vi "AlliGator Calibration Actions.vi"(0 "AlliGator Q Elements":T4[](array[typedef]), 1 "VI in":refnum<vi>, 2 "Script in":bool, 5 "data value reference":refnum<data-value>, 7 "AlliGator Q Event in":T5=enum."GUI:Idle", 9 "Data":variant, 11 "error in (no error)":errorcluster, 12 "AlliGator Ctrl Refnums":T6) -> (3 "Script out":bool, 4 "Alligator Queue Element 1 (+ 2)":T4[](array[typedef]), 6 "AlliGator IV DVR":refnum<data-value>, 10 "[Notebook Message]":T1[](array[typedef]) {"Message Style"."Text Alignment" items=["Left", "Right", "Center"]}, 15 "error out":errorcluster)   [LabVIEW 2021, in "AlliGator Action Engine.lvlib"]
doc: "Processes AlliGator phasor calibration-related actions."
uses:
  AlliGator Action Engine.lvlib
  AlliGator Internal Variables v2.ctl
  <vilib>/vision/Image Controls.llb/IMAQ Image.ctl
  AlliGator Gate Image Set.ctl
  AlliGator FLI Dataset Type.ctl
  AlliGator Data Series Type.ctl
  AlliGator Dataset Channel.ctl
  AlliGator Gate Arithmetic.ctl
  AlliGator Displayed Image.ctl
  Image/Named ROI Description.ctl
  AlliGator Decay Metadata v3.ctl
  AlliGator Decay Background Subtraction Info.ctl
  AlliGator Baseline Subtraction Method.ctl
  Graphs/XY Graph/XY Graph Plot Shift Parameters.ctl
  Graphs/XY Graph/XY Graph Plot Shift Method.ctl
  AlliGator Decay Extrapolation Parameters.ctl
  Phasor/Calibration Phasor (m, phi).ctl
  Phasor/Phasor Reference Series.ctl
  Phasor/Phasor Calibration Map v2.ctl
  Phasor/Phasor (g, s).ctl
  AlliGator Raw Phasor Plot Data v4.ctl
  Phasor/Phasor Standard Deviation Options.ctl
  AlliGator Phasor Multi-Harmonic Data.ctl
  Phasor/Phasor Harmonic Data.ctl
  AlliGator Decay Fit Options & Parameters v2.ctl
  Fits/IRF(X)PSED/Decay Fit Options v2.ctl
  Fits/Decay Convolution/Decay Model.ctl
  Fits/Residual Type.ctl
  Fits/IRF(X)PSED/Fit Weights Type.ctl
  Fits/Non-linear Fitting Method v2.ctl
  Fits/Fit Calculation Method.ctl
  Fits/Non-linear Fitting Algorithm.ctl
  AlliGator Decay Fit Parameter Constraints 2.ctl
  Fits/IRF(X)PSED/Decay Fit Parameters In List.ctl
  Fits/IRF(X)PSED/MLE Baseline Offset Type.ctl
  AlliGator Decay Preprocessing Parameters.ctl
  Fits/IRF(X)PSED/Decay Fit Parameters & Derived Quantities List.ctl
  AlliGator Q Event.ctl
  AlliGator Ctrl Refnums.ctl
  AlliGator Other Ctrl Refnums.ctl
  AlliGator State Indicator.ctl
  AlliGator Phasor Plot Ctrl Refnums.ctl
  AlliGator Phasor Graph Ctrl Refnums.ctl
  Phasor/Phasor Calibration Type.ctl
  AlliGator Dataset Ctrl Refnums.ctl
  AlliGator Registered Events Ctrl Refnums.ctl
  AlliGator Image Histogram Control Refnums.ctl
  Histograms/Linear Histogram Options.ctl
  Histograms/Histogram Bin Option.ctl
  Histograms/Histogram Bin Position.ctl
  AlliGator Decay Fit Map Control Refnums.ctl
  AlliGator Q Element.ctl
  Notebook/Notebook Message Object.ctl
  Rich Text Box/Text Formatting.ctl
  Rich Text Box/Text Colors.ctl
  Alligator Elements Order in Action Stack.ctl
  AlliGator State Indicators List.ctl
  Graphs/XY Graph/XY Graph Mouse Click Event Data.ctl
  Graphs/XY Graph/XY Graph Refnum.ctl
  <vilib>/Utility/miscctls.llb/LVPoint32TypeDef.ctl
  Files/Load-Save File Info.ctl
  c3660eb9-da68-4ace-825a-127935e87b4e.vi
  Variant/Variant to Data/Variant to I32.vi
  Variant/Variant to Data/Variant to Boolean.vi
  AlliGator Add Single Action to Stack.vi
  Graphs/Get Plot at Mouse Click (XY Graph)/Get Plot at Mouse Click [AAC].vi
  AlliGator Add Action Array to Stack.vi
  AlliGator Scripts.lvlib
  GUI/GUI.lvlib
  Phasor/Phasor.lvlib
  AlliGator Settings.lvlib
  AlliGator Phasor Calibration.lvlib
  Files/Files.lvlib
  AlliGator GUI.lvlib
  Rich Text Box/Rich Text Box.lvlib
  Graphs/XY Graph/XY Graph Add-Ons.lvlib
  Graphs/Graphs.lvlib
  AlliGator Phasor Graph.lvlib
  Variant/Variant to Data/Variant to Data.lvlib
  AlliGator Internal Variables.lvlib
  Sound/Sound.lvlib
  AlliGator Source Image.lvlib
  AlliGator Decay Fit Parameter Map.lvlib
  Image/Image.lvlib
  AlliGator Decay Preprocessing.lvlib
  AlliGator Files.lvlib
  AlliGator Phasor Plot.lvlib
  Fits/Fits.lvlib
  AlliGator Decay Fit.lvlib
  AlliGator Dual-Channel Datasets.lvlib
  Histograms/Histogram Window.lvlib
  Notebook/Notebook.lvlib
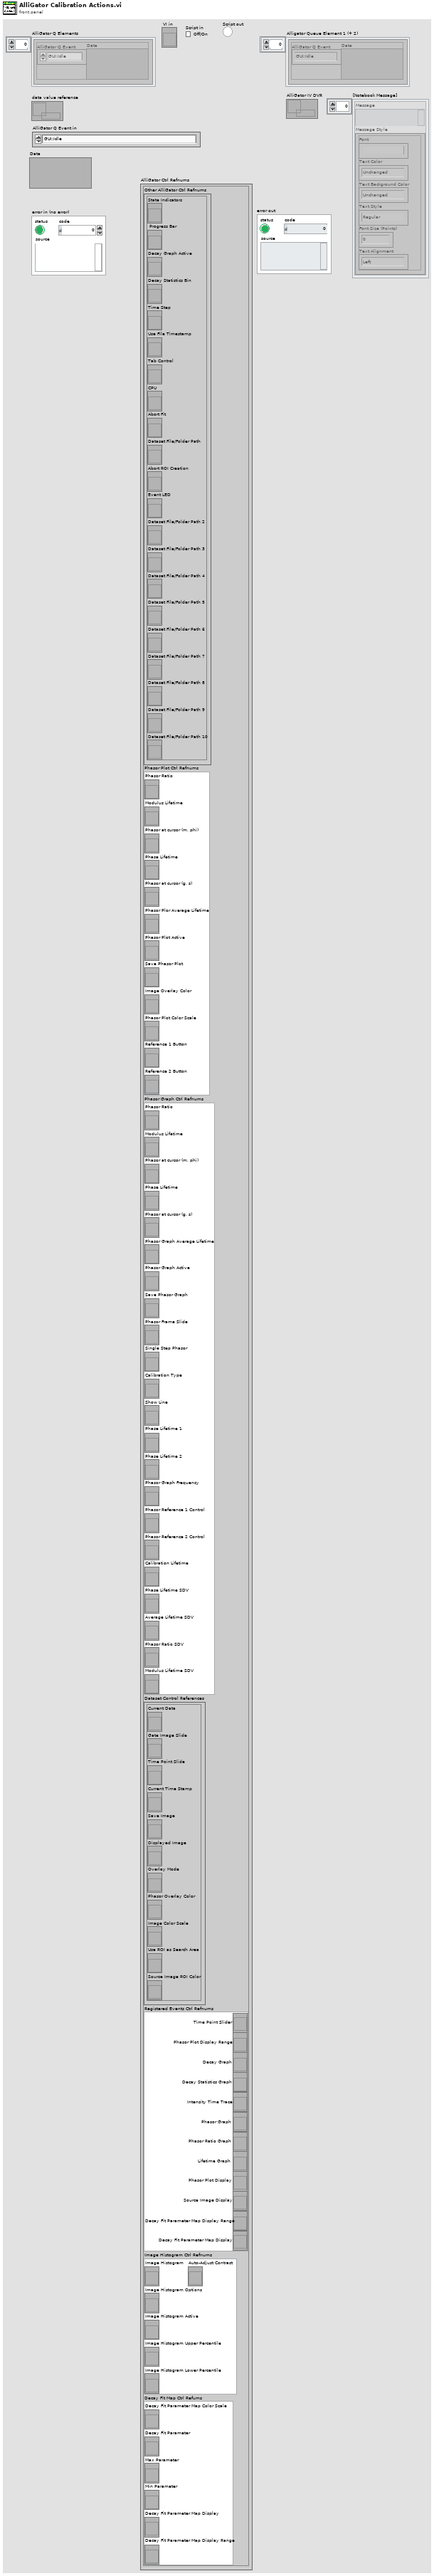
[diagram p1: front panel]
types:
  T1 = typedef "Notebook.lvlib/Notebook Message Object.ctl" = cluster{"Message":string, "Message Style":T2}
  T2 = typedef "Rich Text Box.lvlib/Text Formatting.ctl" = cluster{"Font":string, "Text Color":T3, "Text Background Color":T3, "Text Style":enum16{"Regular", "Bold", "Italic", "Underline", "Strikeout"}, "Font Size (Points)":dbl, "Text Alignment":i32}
  T3 = typedef "Rich Text Box.lvlib/Text Colors.ctl" = enum16{"Unchanged", "Black", "Blue", "Brown", "Gray", "Green", "Orange", "Pink", "Red", "White"}
  T4 = typedef "AlliGator Action Engine.lvlib/AlliGator Q Element.ctl" = cluster{"AlliGator Q Event":T5, "Data":variant}
  T5 = typedef "AlliGator Action Engine.lvlib/AlliGator Q Event.ctl" = enum16{"---- Files ----", "Files:Set Batch Export Files To Save", "Files:Set Dataset Loading & Pre-processing Options", "Files:Check #Frames in Dataset", "Files:Increment Frame Index", "Files:Open Mask Image", "Files:Open White Light Image", "Files:Open Single Dataset", "Files:New Folder of Folders Selected", "Files:Load File (all Types)_Scriptable", "Files:Move Flattened Series to Folders Series", "Files:Select Folder", "Files:Load FLI Dataset", "Files:Load Swiss SPAD 1 Dataset", "Files:Load Swiss SPAD 2 Dataset", "Files:Load .sdt FLI Dataset", "Files:Load .ptu FLI Dataset", "Files:Load .bin FLI Dataset", "Files:Load Single Gate Image Folder", "Files:Load I/m/phi Dataset (deprecated)", "Files:Load Single Image", "Files:Subtract Background File", "Files:Export FLI Dataset", "Files:Load HDF5 FLI Dataset", "Files:Set Destination File Path", "Files:Save Mask Image", "Files:Batch Conversion", "Files:New Folder Selected", "Files:Close FLI Dataset", "Files:Close FLI Dataset Series", "Files:Close White Light Image", "Files:Close Mask Image", "---- FLI Dataset ----", "FLI Dataset:Channel Arithmetic", "FLI Dataset:Export Average Lifetime Map as ASCII", "FLI Dataset:Export User-Defined Quantity Map as ASCII", "FLI Dataset:Python Function FLI Dataset Event", "FLI Dataset:ROI Analysis", "FLI Dataset:Tilted Logistic Square Gated IRF Characteristics Map", "FLI Dataset:Logistic Square Gated IRF Characteristics Map", "FLI Dataset:Square Gated IRF Characteristics Map", "FLI Dataset:Multi-ROI Single-Pixel Phasor Analysis", "FLI Dataset:Multi-ROI Single-Pixel NLSF Analysis", "FLI Dataset:All ROIs IRF Extraction", "FLI Dataset:All ROIs Decay Fit Non-Interactive (Fast + Individual IRF)", "FLI Dataset:All ROIs Phasor Analysis", "FLI Dataset:All ROIs Decay Fit", "FLI Dataset:Fluorescence Decay Statistics", "FLI Dataset:Update Decay Statistics Graph", "FLI Dataset:Get Decay from ROI", "FLI Dataset:All ROIs Average Lifetimes", "---- FLI Dataset Series ----", "FLI Dataset Series:Sum All Datasets in Series", "FLI Dataset Series:Add Dataset to Accumulated Dataset", "FLI Dataset Series:Display Accumulated Dataset", "FLI Dataset Series:Clear Dataset Series Sum", "FLI Dataset Series:Time-Series Analysis (NLSF)", "FLI Dataset Series:Time-Series Analysis (Phasor)", "---- Image ----", "Image:Update Image Profile Plots", "Image:Image Histogram Cursor Move", "Image:Image Histogram", "Image:Image Contrast", "Image:Set Image Histogram Cursor Move Flag", "Image:Clear Image Overlay", "Image:Use ROI as Search Area", "Image:Set ROI Diameter", "Image:Save Image Data as TIFF", "Image:Save Displayed Image with Overlay", "Image:Save Image Overlay Only", "Image:Save Image as Hot Pixel Mask", "Image:Change Source Image Color Palette", "Image:Copy Image to Clipboard", "Image:Source Image ROI Selection", "Image:Delete All ROIs", "Image:Delete All Unselected ROIs", "Image:Delete ROI", "Image:Merge All ROIs", "Image:Store ROI", "Image:Source Image ROI Storage", "Image:Export ROI Description to Notebook", "Image:Save ROI", "Image:Load ROI", "Image:Paste ROI Definition", "Image:Clear ROI", "Image:Identify ROIs in Mask Image", "Image:Create Complementary ROI", "Image:Create Contour ROI", "Image:Create ROI(s) from Pixels with Peak above Min_Scriptable", "Image:Create ROI(s) from Pixels with Intensity above Min_Scriptable", "Image:Compute ROI Statistics", "Image:Delete ROI(s) based on ROI Characteristics", "Image:Create ROI Grid", "Image:ROI to Individual Pixel ROIs", "Image:Python Function Source Image Event", "Image:Show Phasor Calibration Map ROI Centers", "Image:Convert ROI to Mask Image", "Image:Mouse Move", "Image:Mouse Up", "Image:Set Source Image Mouse Move Flag", "Image:Add Scale Bar Overlay", "Image:Delete Existing ROIs Option", "---- Decay ----", "Decay:Clear IRF/Reference Plot", "Decay:Clear Local IRFs", "Decay:Add Decay to Graph", "Decay:Smoothen Plot", "Decay:Smoothen Plot Tail", "Decay:Average Selected Plots", "Decay:Extract IRF", "Decay:Optimal IRF Extraction", "Decay:Threshold IRF", "Decay:Fit to Model IRF", "Decay:Fit IRF to Square Gate", "Decay:Fit IRF to Logistic Square Gate", "Decay:Fit IRF to Tilted Logistic Square Gate", "Decay:Create Bounding Cursors Set", "Decay:Export Bounding Cursors Definition to Notebook", "Decay:Denoise Plot", "Decay:Compute Cumulative Function", "Decay:Use as Reference Decay", "Decay:Show Reference Decay/IRF", "Decay:Extrapolate Decay", "Decay:Create Head & Tail Bounding Cursors", "Decay:Store Cursor-defined Head & Tail Fractions", "Decay:Rebin Plot", "Decay:1-Normalize Decay", "Decay:[0-1]-Normalize Plot", "Decay:Straighten Decay", "Decay:Shift Decay", "Decay:Fold Decay", "Decay:Fit Decay", "Decay:Global Fit of Selected Decays", "Decay:Post Global Fit Script", "Decay:Add Global Fit Parameters to Graph", "Decay:Add Decay Parameter(s) to Plot (Graph)", "Decay:Export Decay to Phasor Graph", "Decay:Plot Decay Shifts", "Decay:Compute Average Lifetime", "Decay:Plot Convolution", "Decay:Graph Tip Strip Update", "---- Decay Statistics ----", "Decay Statistics:Tip Strip Update", "---- Intensity Time Trace ----", "Intensity Time Trace:Use File Timestamp", "Intensity Time Trace:Load Intensity Corrections File", "Intensity Time Trace:Clear Intensity Corrections File", "Intensity Time Trace:Tip Strip Update", "---- Phasor Plot ----", "Phasor Plot:Build Phasor Plot", "Phasor Plot:Change Phasor Plot Color Palette", "Phasor Plot:Adjust Phasor Plot Display Range", "Phasor Plot:Highlight Image ROI in Phasor Plot", "Phasor Plot:Save Phasor Plot Image with Overlay", "Phasor Plot:Export Complex Phasor Map", "Phasor Plot:Export Phasor Ratio Map", "Phasor Plot:Export Average Lifetime Map", "Phasor Plot:Compute Phase Lifetime Histogram", "Phasor Plot:Compute Phasor Ratio Histogram", "Phasor Plot:Compute Phase Lifetime vs Intensity Scatter Plot", "Phasor Plot:Weber 2-Component Decomposition", "Phasor Plot:Update Phasor Color Map Vertices", "Phasor Plot:Clear Phasor Overlay", "Phasor Plot:Use Segment Extremities as References", "Phasor Plot:Use UC/Segment Intersections as References", "Phasor Plot:Use UC/Principal Axis Intersections as References", "Phasor Plot:Use UC/Linear Fit Intersections as References", "Phasor Plot:Update Phasor Plot Reference", "Phasor Plot:Show Local Phasor Info in Phasor Plot", "Phasor Plot:Update Phasor Plot State", "Phasor Plot:Phasor Plot ROI Storage", "Phasor Plot:Phasor Plot ROI Selection", "Phasor Plot:Python Function Phasor Plot Event", "Phasor Plot:Overlay Phasor ROI, Ratio or Map in Source Image", "Phasor Plot:Compute Decay of Selected Phasors", "Phasor Plot:Phasor at Image Pixel", "Phasor Plot:Mouse Move", "Phasor Plot:Mouse Up", "Phasor Plot:Display Range Mouse Move", "Phasor Plot:Set Mouse Move Flag", "---- Phasor Graph ----", "Phasor Graph:Calibrated Phasor Map Series", "Phasor Graph:Whole Image Phasor Scatter Plot (Todo)", "Phasor Graph:Get Phasor Value", "Phasor Graph:Create New Phasor Plot Dialog", "Phasor Graph:Update Last Phasor Value", "Phasor Graph:Update Phasor (m, phi)", "Phasor Graph:Remove Single Phasor from Plot", "Phasor Graph:Add Single Phasor to Plot", "Phasor Graph:Remove Phasor Plot", "Phasor Graph:Remove Selected Phasor Plots", "Phasor Graph:Clear Phasor Data", "Phasor Graph:Clear Phasor Graph", "Phasor Graph:Cursor Move", "Phasor Graph:Draw Cursor Connecting Line", "Phasor Graph:Clear Cursor Connecting Line", "Phasor Graph:Find UC Intersection", "Phasor Graph:Use UC/Cursor-Defined Line Intersections", "Phasor Graph:Use Selected Plots Fitted Line/UC Intersections", "Phasor Graph:Use Selected Plots Principal Axis/UC Intersections", "Phasor Graph:Show Single Phasor", "Phasor Graph:Save Single Phasor Plot", "Phasor Graph:Save All Phasor Plots", "Phasor Graph:Load Phasor Plot(s)", "Phasor Graph:Phasor Multiplication", "Phasor Graph:Compute Average Phasor", "Phasor Graph:Compute Multiple Average Phasors (Selected Plots)", "Phasor Graph:Export Single Phasor Plot Phase Lifetimes", "Phasor Graph:Phase Lifetime Trajectory", "Phasor Graph:Phase Lifetime vs Intensity Scatter Plot (deprecated)", "Phasor Graph:Parameter 2 vs Parameter 1 Scatter Plot", "Phasor Graph:Use Cursor n Location", "Phasor Graph:Set Reference n to Current Phase Lifetime Value", "Phasor Graph:Set Reference n to Lifetime Value", "Phasor Graph:Set Cursor n Location", "Phasor Graph:Save Phasor Graph Image", "Phasor Graph:Update SEPL Plot", "Phasor Graph:Export Single Phasor Plot Data", "Phasor Graph:Export Selected Phasor Plots Data", "Phasor Graph:Python Function Phasor Graph Event", "Phasor Graph:Tip Strip Update", "---- Calibration ----", "Calibration:Set Calibration Type", "Calibration:Load/Save Phasor Calibration", "Calibration:Load/Save Phasor Calibration Series", "Calibration:Load/Save Phasor Calibration Map", "Calibration:Use as Calibration", "Calibration:Compute Optimal Calibration from Phasor References", "Calibration:Clear Phasor Calibration", "Calibration:Single Phasor Calibration Information", "Calibration:Use as Calibration Series", "Calibration:Use as Calibration Map", "Calibration:Clear Calibration Series", "Calibration:Phasor Calibration Series Information", "Calibration:Clear Calibration Map", "Calibration:Phasor Calibration Map Information", "Calibration:Apply Phasor Calibration", "Calibration:Update Single Plot Calibration", "Calibration:Update Multiple Plots Calibration", "Calibration:Clear Single Plot Calibration", "Calibration:Clear All Plots Calibrations", "Calibration:Clear Plot(s) Calibration(s)?", "Calibration:Phasor Calibration Maps (# Gates Series)", "---- Phasor Ratio ----", "Phasor Ratio:Clear Reference n", "Phasor Ratio:Toggle Selected Plot(s)  Lock to Reference 1", "Phasor Ratio:Use as Reference n", "Phasor Ratio:Send Reference n to Notebook", "Phasor Ratio:Toggle Selected Plot(s)  Lock to Reference 2", "Phasor Ratio:Compute Phasor Ratio at Mouse Location", "Phasor Ratio:Compute Phasor Plot's Average Phasor Ratio", "Phasor Ratio:Compute Time-Series Phasor Ratios", "Phasor Ratio:Fit Line to Phasor Ratio Plot", "Phasor Ratio:Save References", "Phasor Ratio:Load References", "Phasor Ratio:Update Phasor Reference 1", "Phasor Ratio:Update Phasor Reference 2", "Phasor Ratio:Move Cursor n to Reference n", "Phasor Ratio:Use as Phasor Reference 1 Lifetime", "Phasor Ratio:Use as Phasor Reference 2 Lifetime", "Phasor Ratio:Export Phasor Ratio Map as ASCII", "Phasor Ratio:Tip Strip Update", "---- Lifetime & Other Parameters Graph ----", "Lifetime:Tip Strip Update", "---- Decay Fit Parameter Map ----", "Decay Fit Parameter Map:Export ROI NLSF Data as ASCII", "Decay Fit Parameter Map:Set Decay Fit  Parameter Map Selection", "Decay Fit Parameter Map:Build Decay Fit Parameter Map", "Decay Fit Parameter Map:Change Decay Fit Parameter Map Color Palette", "Decay Fit Parameter Map:Export Decay Fit Parameter Map Data as ASCII", "Decay Fit Parameter Map:Export All Decay Fit Parameter Maps Data as ASCII", "Decay Fit Parameter Map:Send Map Data to Lifetime Graph", "Decay Fit Parameter Map:Save Decay Fit Parameter Map Image", "Decay Fit Parameter Map:Save-Load IRFs & Fit Data", "Decay Fit Parameter Map:Update Local Decay Plots", "Decay Fit Parameter Map:Python Function Decay Fit Parameters Map Event", "Decay Fit Parameter Map:Overlay Decay Fit Parameter Map in Source Image", "Decay Fit Parameter Map:Plot Map Data vs Intensity", "Decay Fit Parameter Map:Mouse Up", "Decay Fit Parameter Map:Display Range Mouse Move", "---- Generic Graph ----", "Generic Graph:Generic XY Graph Event", "Generic Graph:Python Function XY Graph Event", "Generic Graph:New Plot", "Generic Graph:Save Plot", "Generic Graph:XY Plot Histogram", "Generic Graph:Set XY Graph Plot Name", "Generic Graph:Set Last Cursor Style", "Generic Graph:Tip Strip Update", "---- GUI ----", "GUI:Start Script", "GUI:Type of Displayed Image Changed", "GUI:Gate Image Slide Changed", "GUI:Show Busy Icon", "GUI:Show Busy Icon & Abort Button", "GUI:Hide Busy Icon", "GUI:Hide Busy Icon & Abort Button", "GUI:Abort", "GUI:End Script", "GUI:Start Timing", "GUI:End Timing", "GUI:Set State Indicator", "GUI:Send Parameters JSON Strings to Clipboard", "GUI:Set Gate Step", "GUI:Idle", "GUI:Initialization", "GUI:Quit", "GUI:Increment Dataset Index", "GUI:Set Dataset Index to -1", "GUI:Time Series Slider Moved", "GUI:Time Series Slider Changed", "GUI:Toggle Playback or Loop", "GUI:Playback Script", "GUI:Set Phasor Frequency", "GUI:Open Window", "GUI:Start Test Script", "GUI:End Test Script", "DEBUG"}
  T6 = typedef "AlliGator GUI.lvlib/AlliGator Ctrl Refnums.ctl" = cluster{"Other AlliGator Ctrl Refnums":T7, "Phasor Plot Ctrl Refnums":T8, "Phasor Graph Ctrl Refnums":T9, "Dataset Control References":T10, "Registered Events Ctrl Refnums":T11, "Image Histogram Ctrl Refnums":T12, "Decay Fit Map Ctrl Refums":T13}
  T7 = typedef "AlliGator GUI.lvlib/AlliGator Other Ctrl Refnums.ctl" = cluster{"State Indicators":refnum<vi>, " Progress Bar":refnum<vi>, "Decay Graph Active":refnum<vi>, "Decay Statistics Bin":refnum<vi>, "Time Step":refnum<vi>, "Use File Timestamp":refnum<vi>, "Tab Control":refnum<vi>, "CPU":refnum<vi>, "Abort Fit":refnum<vi>, "Dataset File/Folder Path":refnum<vi>, "Abort ROI Creation":refnum<vi>, "Event LED":refnum<vi>, "Dataset File/Folder Path 2":refnum<vi>, "Dataset File/Folder Path 3":refnum<vi>, "Dataset File/Folder Path 4":refnum<vi>, "Dataset File/Folder Path 5":refnum<vi>, "Dataset File/Folder Path 6":refnum<vi>, "Dataset File/Folder Path 7":refnum<vi>, "Dataset File/Folder Path 8":refnum<vi>, "Dataset File/Folder Path 9":refnum<vi>, "Dataset File/Folder Path 10":refnum<vi>}
  T8 = typedef "AlliGator GUI.lvlib/AlliGator Phasor Plot Ctrl Refnums.ctl" = cluster{"Phasor Ratio":refnum<vi>, "Modulus Lifetime":refnum<vi>, "Phasor at cursor (m, phi)":refnum<vi>, "Phase Lifetime":refnum<vi>, "Phasor at cursor (g, s)":refnum<vi>, "Phasor Plor Average Lifetime":refnum<vi>, "Phasor Plot Active":refnum<vi>, "Save Phasor Plot":refnum<vi>, "Image Overlay Color":refnum<vi>, "Phasor Plot Color Scale":refnum<vi>, "Reference 1 Button":refnum<vi>, "Reference 2 Button":refnum<vi>}
  T9 = typedef "AlliGator GUI.lvlib/AlliGator Phasor Graph Ctrl Refnums.ctl" = cluster{"Phasor Ratio":refnum<vi>, "Modulus Lifetime":refnum<vi>, "Phasor at cursor (m, phi)":refnum<vi>, "Phase Lifetime":refnum<vi>, "Phasor at cursor (g, s)":refnum<vi>, "Phasor Graph Average Lifetime":refnum<vi>, "Phasor Graph Active":refnum<vi>, "Save Phasor Graph":refnum<vi>, "Phasor Frame Slide":refnum<vi>, "Single Step Phasor":refnum<vi>, "Calibration Type":refnum<vi>, "Show Line":refnum<vi>, "Phase Lifetime 1":refnum<vi>, "Phase Lifetime 2":refnum<vi>, "Phasor Graph Frequency":refnum<vi>, "Phasor Reference 1 Control":refnum<vi>, "Phasor Reference 2 Control":refnum<vi>, "Calibration Lifetime":refnum<vi>, "Phase Lifetime SDV":refnum<vi>, "Average Lifetime SDV":refnum<vi>, "Phasor Ratio SDV":refnum<vi>, "Modulus Lifetime SDV":refnum<vi>}
  T10 = typedef "AlliGator GUI.lvlib/AlliGator Dataset Ctrl Refnums.ctl" = cluster{"Current Data":refnum<vi>, "Gate Image Slide":refnum<vi>, "Time Point Slide":refnum<vi>, "Current Time Stamp":refnum<vi>, "Save Image":refnum<vi>, "Displayed Image":refnum<vi>, "Overlay Mode":refnum<vi>, "Phasor Overlay Color":refnum<vi>, "Image Color Scale":refnum<vi>, "Use ROI as Search Area":refnum<vi>, "Source Image ROI Color":refnum<vi>}
  T11 = typedef "AlliGator GUI.lvlib/AlliGator Registered Events Ctrl Refnums.ctl" = cluster{"Time Point Slider":refnum<vi>, "Phasor Plot Display Range":refnum<vi>, "Decay Graph":refnum<vi>, "Decay Statistics Graph":refnum<vi>, "Intensity Time Trace":refnum<vi>, "Phasor Graph":refnum<vi>, "Phasor Ratio Graph":refnum<vi>, "Lifetime Graph":refnum<vi>, "Phasor Plot Display":refnum<vi>, "Source Image Display":refnum<vi>, "Decay Fit Parameter Map Display Range":refnum<vi>, "Decay Fit Parameter Map Display":refnum<vi>}
  T12 = typedef "AlliGator GUI.lvlib/AlliGator Image Histogram Control Refnums.ctl" = cluster{"Image Histogram":refnum<vi>, "Image Histogram Options":refnum<vi>, "Image Histogram Active":refnum<vi>, "Image Histogram Upper Percentile":refnum<vi>, "Image Histogram Lower Percentile":refnum<vi>, "Auto-Adjust Contrast":refnum<vi>}
  T13 = typedef "AlliGator Decay Fit Parameter Map.lvlib/AlliGator Decay Fit Map Control Refnums.ctl" = cluster{"Decay Fit Parameter Map Color Scale":refnum<vi>, "Decay Fit Parameter":refnum<vi>, "Max Parameter":refnum<vi>, "Min Parameter":refnum<vi>, "Decay Fit Parameter Map Display":refnum<vi>, "Decay Fit Parameter Map Display Range":refnum<vi>}
  T14 = typedef "AlliGator Action Engine.lvlib/Alligator Elements Order in Action Stack.ctl" = enum16{"Enqueue 2 AFTER 1", "Enqueue 2 BEFORE 1"}
  T15 = typedef "AlliGator Action Engine.lvlib/AlliGator State Indicators List.ctl" = enum16{"Phasor Calibration Defined", "Phasor Calibration Series Defined", "Phasor Calibration Map Defined", "Phasor Reference 1 Defined", "Phasor Reference 2 Defined", "Lifetime Reference 1 Defined", "Lifetime Reference 2 Defined", "Phasor Calibration Used", "Phasor Calibration Series Used", "Phasor Calibration Map Used", "Dataset Update Needed", "Phasor Plot Update Needed", "Reference/IRF Defined", "Individual IRFs Defined"}
  T16 = typedef "Phasor.lvlib/Phasor Calibration Map v2.ctl" = cluster{"Phasor Frequency":dbl[unit], "Calibration Lifetime":dbl[unit], "ROI Centers":cluster{"X":i32, "Y":i32}[], "ROI Descriptors":T17[], "Map Resolution X":i32, "Map Resolution Y":i32, "z Array":cdb[]}
  T17 = typedef "ROI Descriptor" = cluster{"Global Rectangle":i32[], "Contours":cluster{"ID":enum32{"External", "Internal"}, "Type":u32, "Coordinates":i32[]}[]}
  T18 = typedef "Phasor.lvlib/Phasor Reference Series.ctl" = cluster{"m Array":dbl[], "phi Array":dbl[], "Phasor Frequency":dbl[unit], "Calibration Lifetime":dbl[unit]}
  T19 = typedef "Phasor.lvlib/Calibration Phasor (m, phi).ctl" = cluster{"m":dbl, "phi":dbl, "Phasor Frequency":dbl[unit], "Reference Lifetime":dbl[unit]}
  T20 = typedef "XY Graph Add-Ons.lvlib/XY Graph Mouse Click Event Data.ctl" = cluster{"Multiplot XY Graph":T21, "Mouse Coordinates":T22}
  T21 = typedef "XY Graph Add-Ons.lvlib/XY Graph Refnum.ctl" = refnum<vi>
  T22 = typedef "LVPoint32TypeDef.ctl" = cluster{"Horizontal":i32, "Vertical":i32}
  T23 = typedef "Files.lvlib/Load-Save File Info.ctl" = cluster{"Load/Save":bool, "File Path":path}
  T24 = typedef "Phasor.lvlib/Phasor Calibration Type.ctl" = enum16{"None", "Single Phasor", "Phasor Series", "Phasor Map"}
  T25 = typedef "Phasor.lvlib/Phasor (g, s).ctl" = cluster{"g":dbl, "s":dbl}
  T26 = typedef "AlliGator Internal Variables.lvlib/AlliGator Internal Variables v2.ctl" = cluster{"Displayed Image":T27, "White Light Image":T27, "Mask Image":T27, "ROI Mask Image":T27, "Current Dataset Images 1":T28, "Background Dataset Images 1":T28, "Current Dataset Images 2":T28, "Background Dataset Images 2":T28, "Current Dataset Arithmetic Images":T28, "Accumulated Dataset Images 1":T28, "Accumulated Dataset Images 2":T28, "Accumulated Dataset Arithmetic Images":T28, "Phasor Plot Image":T27, "Decay Fit Parameter Map Image":T27, "Single Data Point Path":path, "White Light Image Path":path, "Mask Image Path":path, "Time-Series Folder":path, "[Time-Series Paths]":path[], "Current Dataset":i32, "Single Dataset Type":T29, "Current Folder":string, "AlliGator Data Series Type":T30, "# Datasets":i32, "Dual-Channel Dataset":bool, "Selected Channel Name":string, "Dataset Channel":T31, "Channel Arithmetic":T32, "Dual-Channel Background Dataset":bool, "Background Channel":T31, "Dual-Channel Accumulated Dataset":bool, "Start Time":dbl, "[Time-Series Timestamps]":dbl[], "[Intensity Corrections]":dbl[], "Time Series Script":bool, "Type of Displayed Image":T33, "Gate Image Slide":u16, "# Gates":i32, "ROIs":T34[], "ROI Decay":cluster{"t Array":dbl[], "I Array":dbl[]}, "Valid Decay":bool, "Decay  Metadata":T35, "Reference Decay Plot Name":string, "Reference Decay":cluster{"t Array":dbl[], "I Array":dbl[]}, "Decay Shift Plot":cluster{"Time Stamps":dbl[], "Decay Shifts":dbl[]}, "[Decays Max Values]":sgl[], "[Decays Min Values]":sgl[], "Calibration Phasor":T19, "Calibration Phasor Series":T18, "Phasor Calibration Map":T16, "Calibration Map MD5 Digest":string, "Last Raw Phasor":T25, "Last Calibrated Phasor":T25, "Last Calibrated Phasor SDV":T25, "Phasor Graph:Phasor Plot":cluster{"g Array":dbl[], "s Array":dbl[]}, "Phasor Graph:Phasor SDV Plot":cluster{"g Array":dbl[], "s Array":dbl[]}, "[Phasor Graph:Raw Phasor Plots]":T41[], "Phasor Plot locked to Ref 1":i32, "[Phasor Plot(s) locked to Ref 1]":i32[], "[Phasor Plot(s) locked to Ref 2]":i32[], "[Pixel Phasors]":T25[], "[[Sum Image]]":dbl[][], "[[CSG Phasors]]":csg[][], "[[Valid Pixel?]]":bool[][], "I/m/phi Dataset":cluster{"I/m/phi Dataset?":bool, "Base Frequency":dbl[unit], "Harmonic Orders":u8[]}, "Multi Phasor Plot Data":T43, "Decay Fit Options & Parameters":T45, "Fit Options: Decay Preprocessing Parameters":T56, "Fit Options: Reference Decay":cluster{"t Array":dbl[], "I Array":dbl[]}, "Is Full Image Parameters Map":bool, "Is Single-Pixels Parameters Map":bool, "NLSF Parameters Map X Resolution":i32, "NLSF Parameters Map Y Resolution":i32, "[Single Decay Fit Parameters]":dbl[], "Fit Model":T47, "[[Multiple Decays Fit Parameters]]":dbl[][], "[[Multiple Decays Fit Parameter SDVs]]":dbl[][], "[[IRFs]]":dbl[][], "IRF Array Time Axis":dbl[], "Decay Array Time Axis":dbl[], "[Decay Fit Parameter Names]":T57[], "[[Phasor Ratios]]":dbl[][], "[[Average Lifetimes]]":dbl[][], "Amplitude Weighted Average Lifetime":bool, "[Decay Sum]":dbl[], "[[User-defined Quantities]]":dbl[][], "User-defined Quantity":string}
  T27 = typedef "IMAQ Image.ctl" = refnum<image>
  T28 = typedef "AlliGator Internal Variables.lvlib/AlliGator Gate Image Set.ctl" = cluster{"SGL Image Max":T27, "SGL Image Sum":T27, "SGL Gate Images":T27[], "SGL Image Min":T27}
  T29 = typedef "AlliGator Files.lvlib/AlliGator FLI Dataset Type.ctl" = enum16{"HDF5 FLI Dataset", "Gate Image Folder", ".sdt FLI Dataset (Becker & Hickl)", ".ptu FLI Dataset (PicoQuant)", "SS1 FLI Dataset", "SS2 FLI Dataset", "I/m/phi Dataset", ".bin FLI Dataset (PicoQuant Binned)", ".bin FLI Dataset (Piccolo Binned)"}
  T30 = typedef "AlliGator Files.lvlib/AlliGator Data Series Type.ctl" = enum16{"Not a Supported Series", "Gate Images Folder Series", "SwissSPAD 2 Dataset Series", "B&H FLI Dataset Series", "PicoQuant PTU FLI Dataset Series", "PicoQuant BIN FLI Dataset Series", "Piccolo hist BIN FLI Dataset Series", "HDF5 FLI Dataset Series"}
  T31 = typedef "AlliGator Dual-Channel Datasets.lvlib/AlliGator Dataset Channel.ctl" = enum16{"G2", "INT"}
  T32 = typedef "AlliGator Settings.lvlib/AlliGator Gate Arithmetic.ctl" = enum16{"None", "INT-G2", "G2/INT*<INT>", "(1 - G2/INT)*<INT>"}
  T33 = typedef "AlliGator Source Image.lvlib/AlliGator Displayed Image.ctl" = enum16{"Single Gate", "Sum of All Gates", "Max of All Gates", "Min of All Gates", "-", "White Ligth Image", "Mask Image"}
  T34 = typedef "Image.lvlib/Named ROI Description.ctl" = cluster{"ROI Descriptor":T17, "ROI Name":string, "Overlay Color":u32}
  T35 = typedef "AlliGator Phasor Graph.lvlib/AlliGator Decay Metadata v3.ctl" = cluster{"ROI Descriptor":T17, "ROI Center":cluster{"X":i32, "Y":i32}, "Decay Background Subtraction Info":T36, "Decay Reverted":bool, "Decay Smoothened":bool, "Decay Straightened":bool, "Fitted Tau (Decay Straightening)":dbl, "Decay Shift Parameters":T38, "Decay Shifted":bool, "Decay Extrapolated":bool, "Decay Extrapolation Parameters":T40, "Decay Normalized":bool, "Fold Decay":bool, "# Folds":u32}
  T36 = typedef "AlliGator Decay Analysis.lvlib/AlliGator Decay Preprocessing.lvlib/AlliGator Decay Background Subtraction Info.ctl" = cluster{"Laser Period":dbl[unit], "Gate Duration":dbl[unit], "Baseline Subtraction Method":T37, "Background Definition Range":cluster{"Min Gate":dbl[unit], "Max Gate":dbl[unit]}, "Total Intensity w/o Bkgd Subtraction":dbl, "Bkgd-subtracted Intensity (exp)":dbl, "# Data Points":i32, "Background/Gate":dbl, "Fitted Lifetime":dbl[unit], "Bkgd-subtracted Intensity (theo)":dbl}
  T37 = typedef "AlliGator Decay Analysis.lvlib/AlliGator Decay Preprocessing.lvlib/AlliGator Baseline Subtraction Method.ctl" = enum16{"Mean", "Min", "Square Gated Single-Exponential", "File", "Constant"}
  T38 = typedef "XY Graph Add-Ons.lvlib/XY Graph Plot Shift Parameters.ctl" = cluster{"Type":T39, "Shift":dbl[unit], "Threshold":dbl, "Rotate":bool}
  T39 = typedef "XY Graph Add-Ons.lvlib/XY Graph Plot Shift Method.ctl" = enum16{"Default", "CFD", "Threshold", "Cross-Correlation"}
  T40 = typedef "AlliGator Decay Analysis.lvlib/AlliGator Decay Preprocessing.lvlib/AlliGator Decay Extrapolation Parameters.ctl" = cluster{"Additional Points":u32, "Head Fraction":dbl, "Fitted Tau":dbl, "Use Periodicity":bool, "Use Cursors":bool, "Tail Fraction":dbl}
  T41 = typedef "AlliGator Phasor Graph.lvlib/AlliGator Raw Phasor Plot Data v4.ctl" = cluster{"Phasor Plot Name":string, "Raw Phasor Plot":T25[], "Phasor Frequency":dbl[unit], "[Decay Metadata]":T35[], "Raw Phasor Plot SDV":T25[], "Phasor SDV Options":T42, "[Calibration Phasor]":T19[]}
  T42 = typedef "Phasor.lvlib/Phasor Standard Deviation Options.ctl" = cluster{"Compute Estimated SDV":bool, "# Replicas":u32, "Use Estimated Average Phasor":bool}
  T43 = typedef "AlliGator Phasor Plot.lvlib/AlliGator Phasor Multi-Harmonic Data.ctl" = cluster{"Base Frequency":dbl[unit], "# Harmonics":u8, "Harmonic Orders":u8[], "Phasor Plot Settings Checksum":u64, "Phasor Harmonic Data Array":T44[]}
  T44 = typedef "Phasor.lvlib/Phasor Harmonic Data.ctl" = cluster{"Phasor Harmonic Name":string, "Phasor Plot Settings Checksum":u64, "Phasor Frequency":dbl[unit], "Base Frequency":dbl[unit], "Harmonic Order":u8, "Phasor Plot Parameters":string, "Phasor Array [[CSG]]":csg[][], "Dataset File Path":path}
  T45 = typedef "AlliGator Decay Fit Parameter Map.lvlib/AlliGator Decay Fit Options & Parameters v2.ctl" = cluster{"SYNC Period":dbl[unit], "Fit Options":T46, "Fit Parameter Constraints":T53[], "MLE Baseline Offset":dbl, "MLE Baseline Offset Type":T55}
  T46 = typedef "Fits.lvlib/Decay Fit Options v2.ctl" = cluster{"Show Fit Residuals":bool, "Fit Model":T47, "Residual Type":T48, "Max Decay Percentile":dbl, "Min Decay Percentile":dbl, "Show Full Decay":bool, "Weights":T49, "Fitting Method":T50, "Compute Parameter Uncertainties":bool, "Periodic Boundaries":bool, "Model Calculation":T51, "Period":dbl[unit], "Termination Criteria":cluster{"Max Iterations":i32, "Max Function Calls":i32, "Max Time":dbl[unit], "Function Tolerance":dbl, "Parameter Tolerance":dbl, "Gradient Tolerance":dbl, "Min Lambda":dbl, "Max Lambda":dbl, "Initial Tick Count":u32}, "Offset Resolution":dbl[unit], "Use Local IRF":bool, "Fitting Algorithm":T52}
  T47 = typedef "Fits.lvlib/Decay Model.ctl" = enum16{"1-Exponential", "2-Exponentials"}
  T48 = typedef "Fits.lvlib/Residual Type.ctl" = enum16{"Standard", "Normalized", "Reduced"}
  T49 = typedef "Fits.lvlib/Fit Weights Type.ctl" = enum16{"Unweighted", "1/Variance", "Best of All"}
  T50 = typedef "Fits.lvlib/Non-linear Fitting Method v2.ctl" = enum16{"Least Square", "Least Absolute Residual", "Bisquare", "MLE", "-", "Best of All"}
  T51 = typedef "Fits.lvlib/Fit Calculation Method.ctl" = enum16{"Simulation", "Convolution", "Integration"}
  T52 = typedef "Fits.lvlib/Non-linear Fitting Algorithm.ctl" = enum16{"Levenberg-Marquardt", "Trust-Region Dogleg"}
  T53 = typedef "AlliGator Decay Analysis.lvlib/AlliGator Decay Fit.lvlib/AlliGator Decay Fit Parameter Constraints 2.ctl" = cluster{"Fit Parameter":T54, "Min Value":dbl, "Max Value":dbl, "Global":bool, "Used":bool}
  T54 = typedef "Fits.lvlib/Decay Fit Parameters In List.ctl" = enum16{"Offset", "Baseline", "A_1", "tau_1", "A_2", "tau_2"}
  T55 = typedef "Fits.lvlib/MLE Baseline Offset Type.ctl" = enum32{"Absolute", "Percentage"}
  T56 = typedef "AlliGator Decay Analysis.lvlib/AlliGator Decay Preprocessing.lvlib/AlliGator Decay Preprocessing Parameters.ctl" = cluster{"Background Subtraction":bool, "Straighten Decay":bool, "Reverse Gates":bool, "1-Normalized Decay":bool, "Smoothen Decay":bool, "Smoothing Parameter":dbl, "Shift Decay":bool, "Decay Shift Parameters":T38, "Extrapolate Decay":bool, "Additional Points":u32, "Head Fraction":dbl, "Pixel-Normalize Decay":bool, "Use Periodicity":bool, "Use Cursors":bool, "Tail Fraction":dbl, "Use Decay Pre-Processing":bool, "Fold Decay":bool, "# Folds":u32, "[0-1]-Normalized Decay":bool}
  T57 = typedef "Fits.lvlib/Decay Fit Parameters & Derived Quantities List.ctl" = enum16{"Offset", "Baseline", "A_1", "tau_1", "A_2", "tau_2", "<tau>_a", "f1_a", "f2_a", "<tau>_i", "f1_i", "f2_i", "-", "R^2", "Chi^2"}
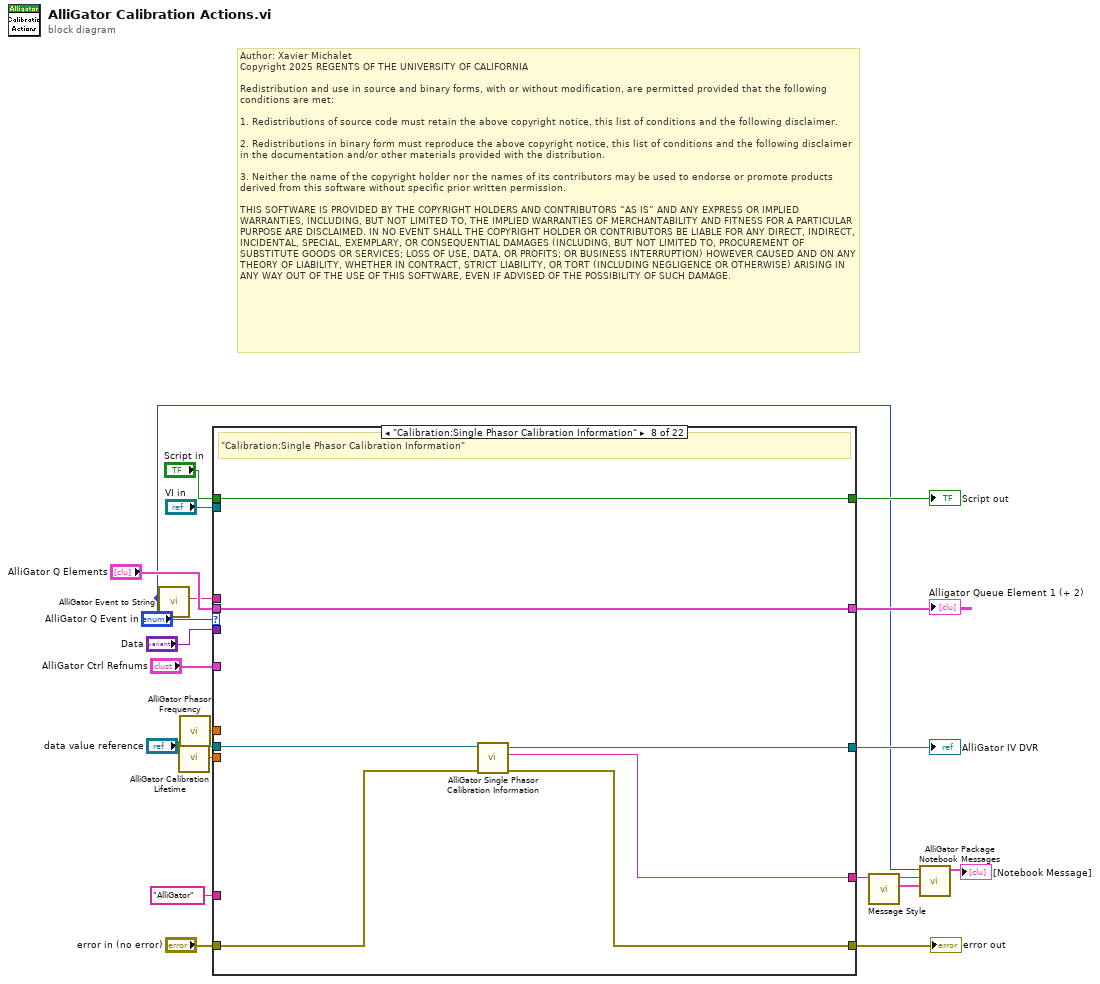
[diagram p0: block diagram]
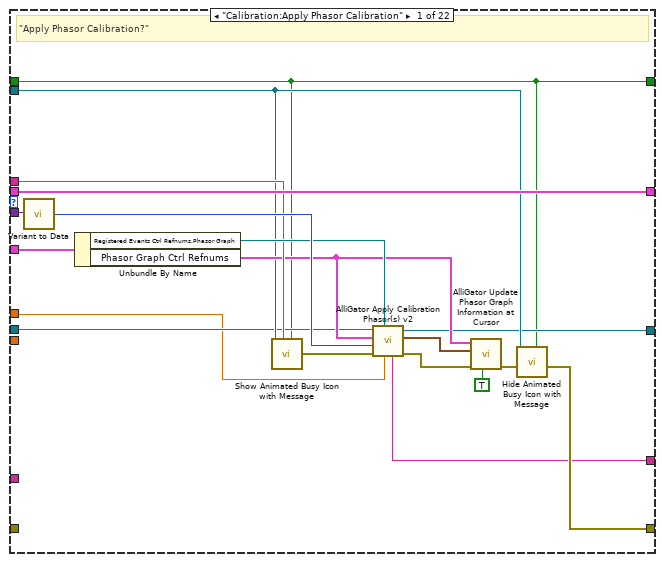
[diagram p2: hidden frame]
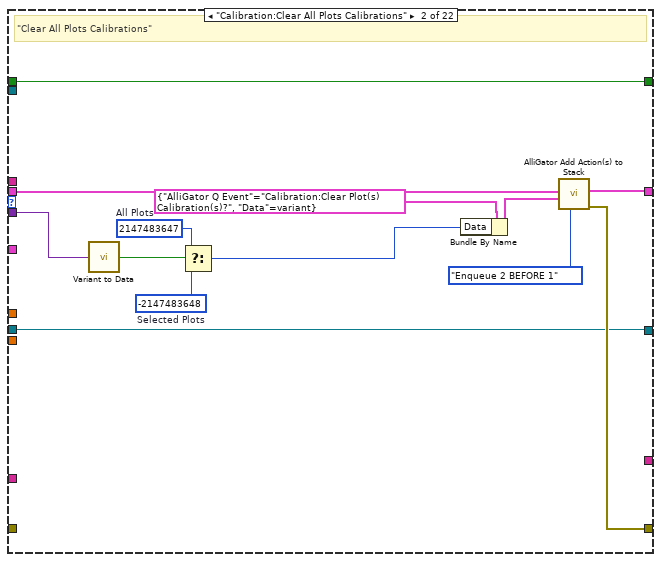
[diagram p3: hidden frame]
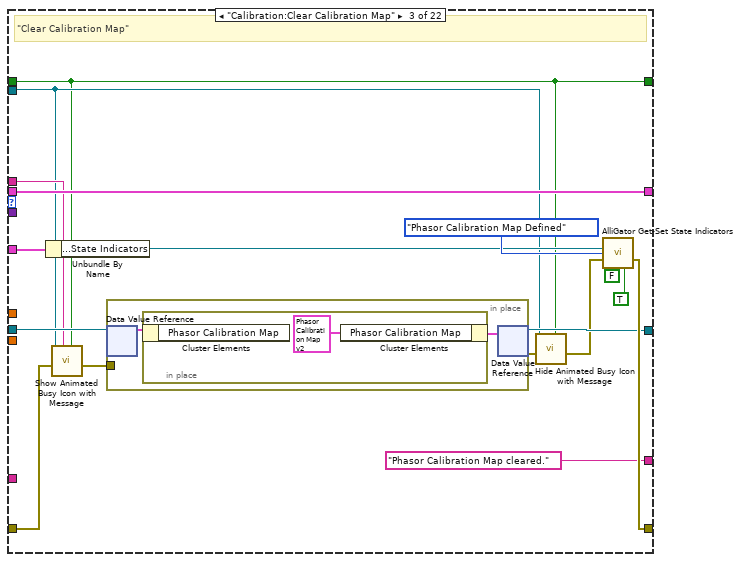
[diagram p4: hidden frame]
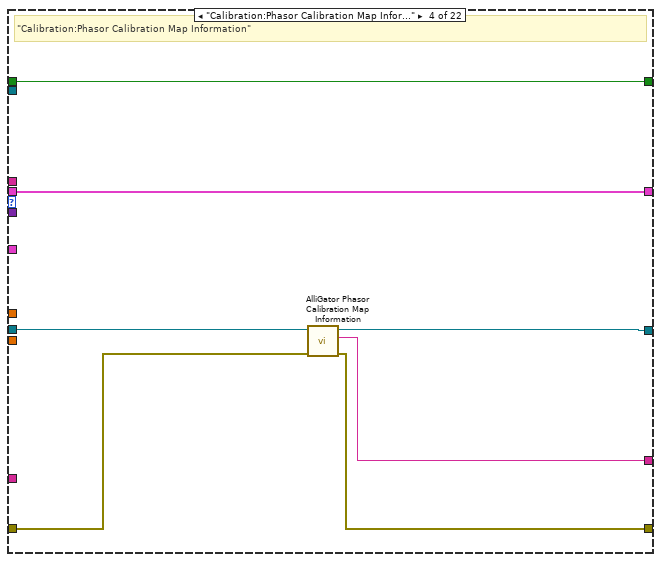
[diagram p5: hidden frame]
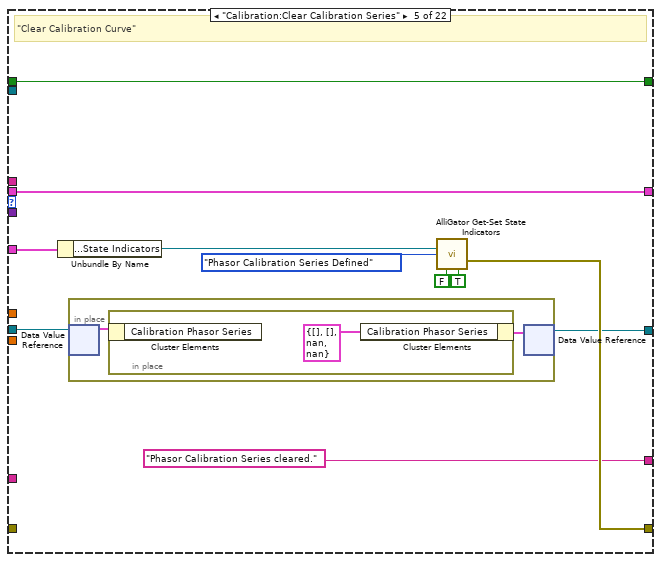
[diagram p6: hidden frame]
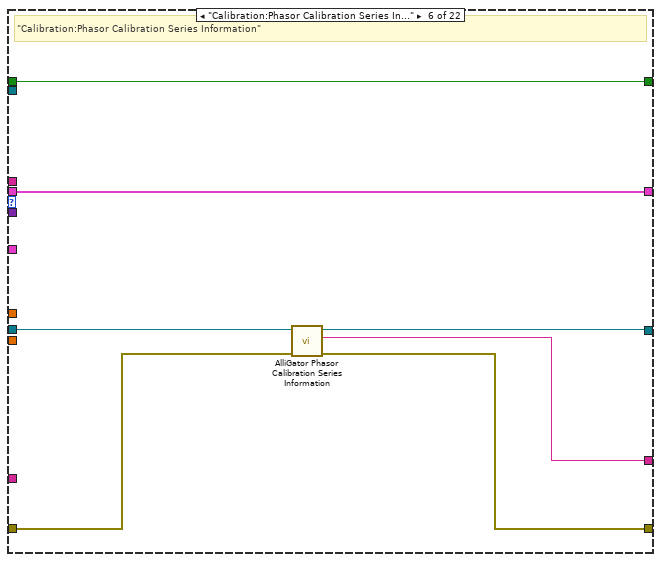
[diagram p7: hidden frame]
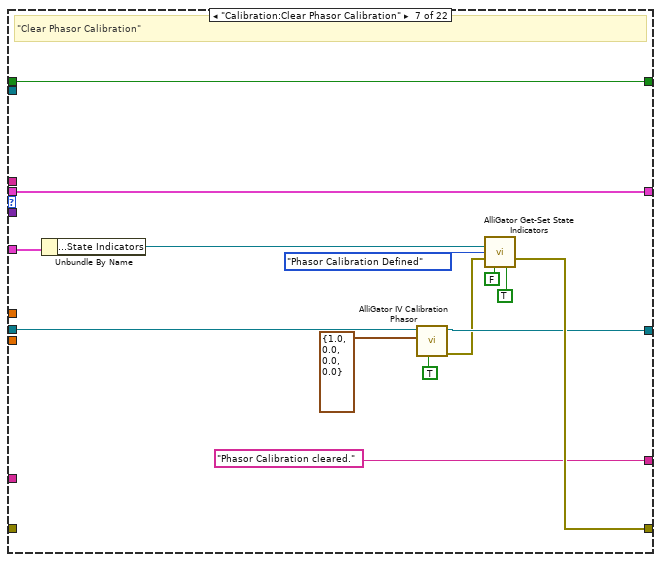
[diagram p8: hidden frame]
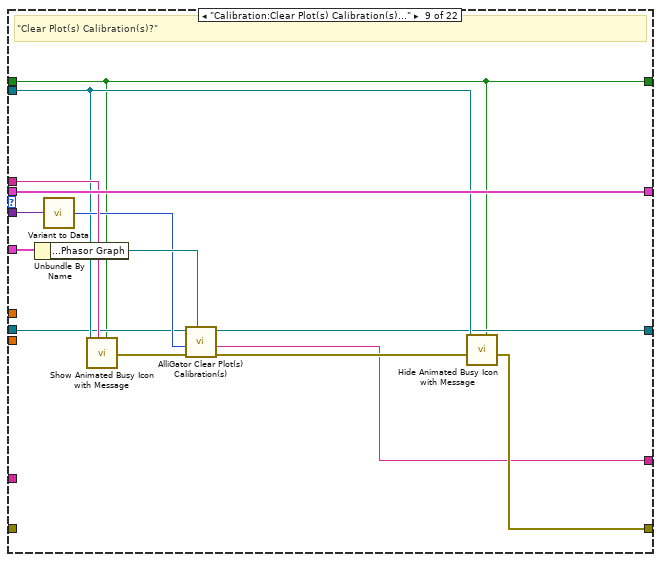
[diagram p9: hidden frame]
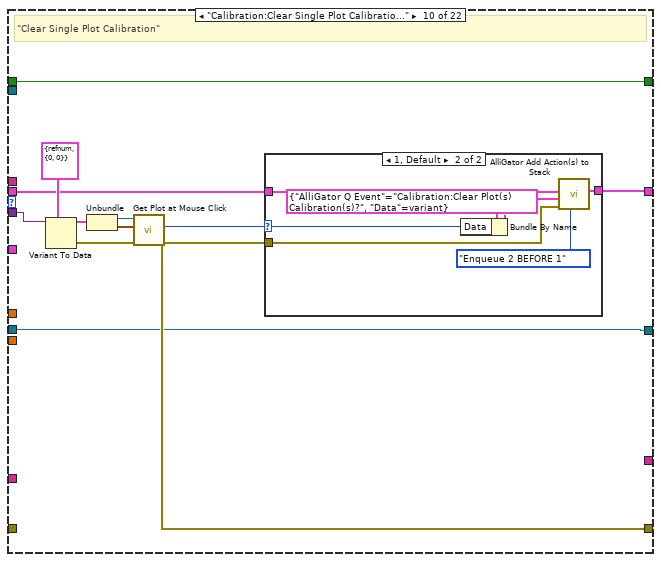
[diagram p10: hidden frame]
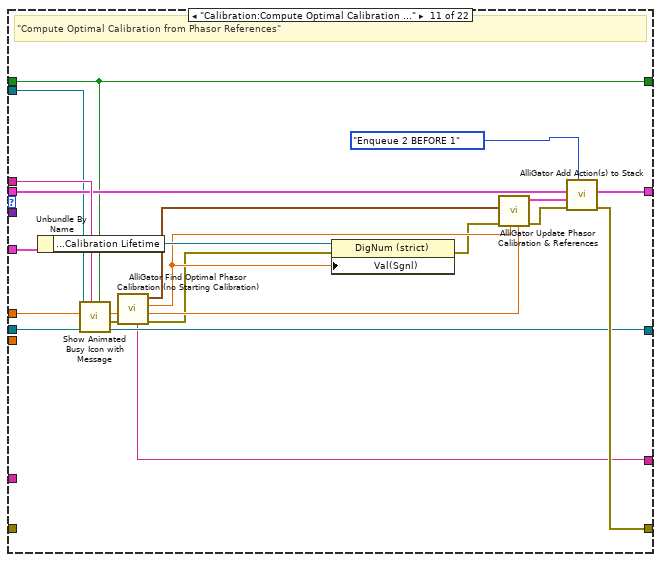
[diagram p12: hidden frame]
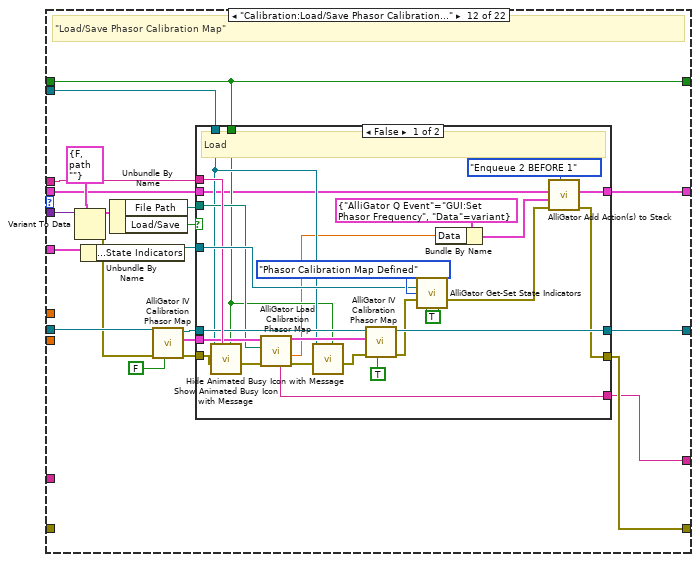
[diagram p13: hidden frame]
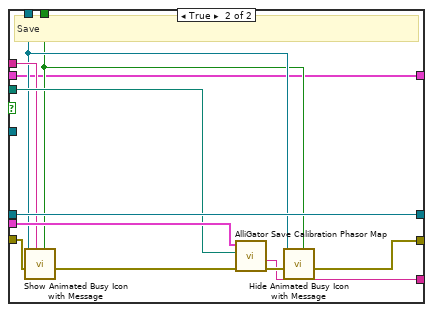
[diagram p14: hidden frame]
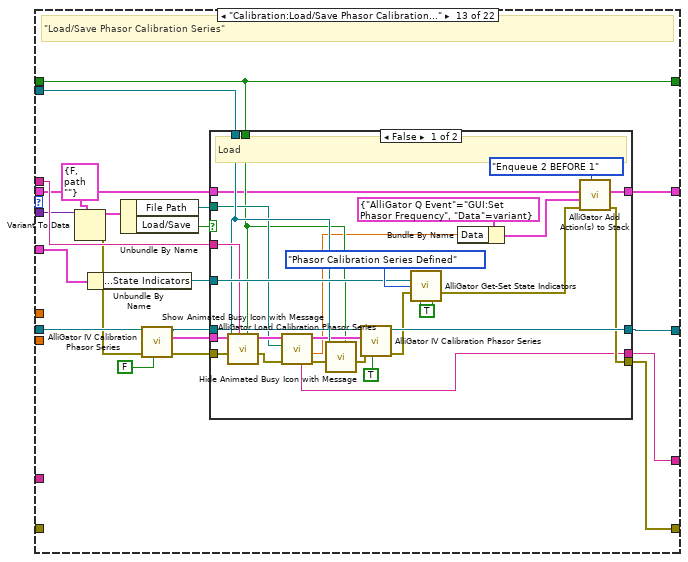
[diagram p15: hidden frame]
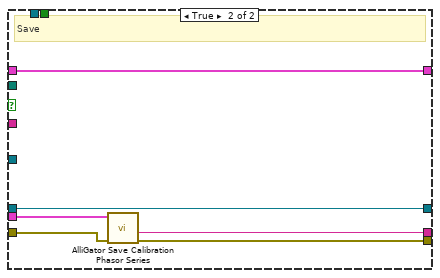
[diagram p16: hidden frame]
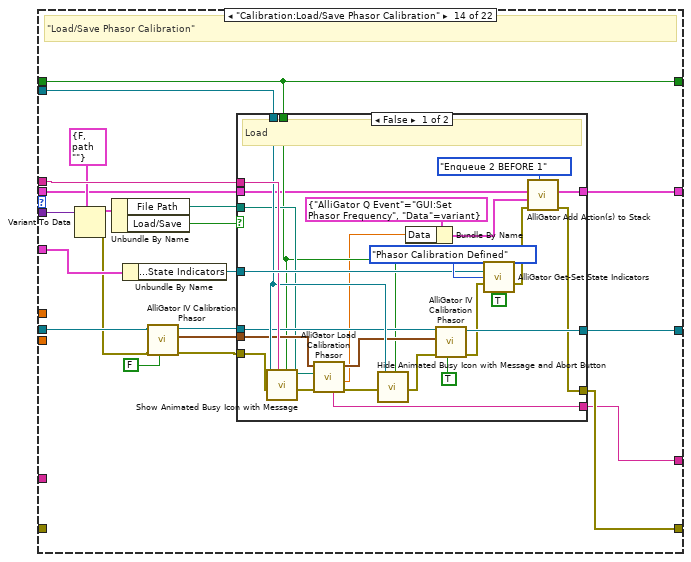
[diagram p17: hidden frame]
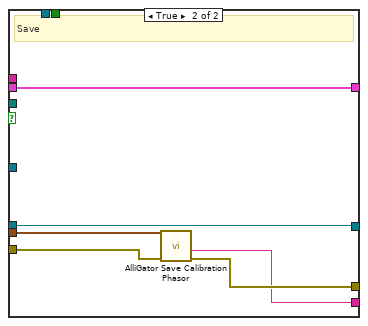
[diagram p18: hidden frame]
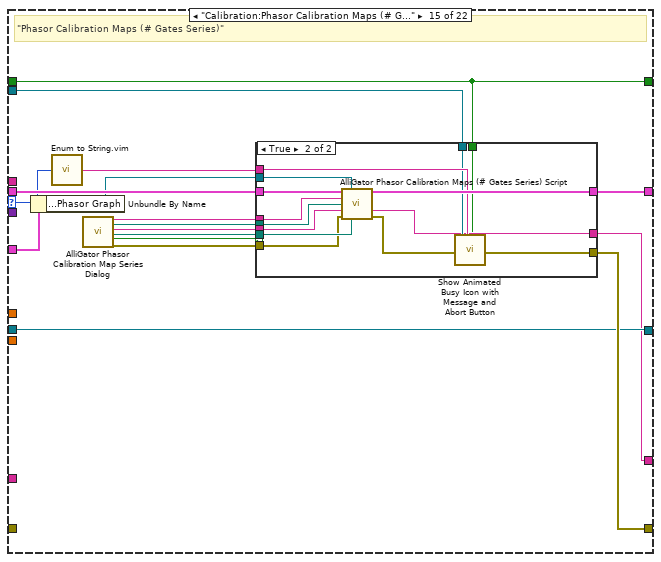
[diagram p19: hidden frame]
diagram:
  # "Author: Xavier Michalet\nCopyright 2025 REGENTS OF THE UNIVERSITY OF CALIFORNIA\n\nRedistribution and use in source and binary forms, with or without modification, are permitted provided that the following conditions are met:\n\n1. Redistributions of source code must retain the above copyright notice, this list of conditions and the following disclaimer.\n\n2. Redistributions in binary form must reproduce the above copyright notice, this list of conditions and the following disclaimer in the documentation and/or other materials provided with the distribution.\n\n3. Neither the name of the copyright holder nor the names of its contributors may be used to endorse or promote products derived from this software without specific prior written permission.\n\nTHIS SOFTWARE IS PROVIDED BY THE COPYRIGHT HOLDERS AND CONTRIBUTORS “AS IS” AND ANY EXPRESS OR IMPLIED WARRANTIES, INCLUDING, BUT NOT LIMITED TO, THE IMPLIED WARRANTIES OF MERCHANTABILITY AND FITNESS FOR A PARTICULAR PURPOSE ARE DISCLAIMED. IN NO EVENT SHALL THE COPYRIGHT HOLDER OR CONTRIBUTORS BE LIABLE FOR ANY DIRECT, INDIRECT, INCIDENTAL, SPECIAL, EXEMPLARY, OR CONSEQUENTIAL DAMAGES (INCLUDING, BUT NOT LIMITED TO, PROCUREMENT OF SUBSTITUTE GOODS OR SERVICES; LOSS OF USE, DATA, OR PROFITS; OR BUSINESS INTERRUPTION) HOWEVER CAUSED AND ON ANY THEORY OF LIABILITY, WHETHER IN CONTRACT, STRICT LIABILITY, OR TORT (INCLUDING NEGLIGENCE OR OTHERWISE) ARISING IN ANY WAY OUT OF THE USE OF THIS SOFTWARE, EVEN IF ADVISED OF THE POSSIBILITY OF SUCH DAMAGE."
  n1 = call "AlliGator Event to String.vi"("AlliGator Q Event"="AlliGator Q Event in") -> ("String"=w6:string)  [unwired: 8 in]
  n2 = call "AlliGator Calibration Lifetime.vi"() -> ("Calibration Lifetime"=w17:dbl[unit])
  n3 = call "AlliGator Phasor Frequency.vi"() -> ("Phasor Frequency"=w12:dbl[unit])
  n4 = case shown="\"Calibration:Single Phasor Calibration Information\"" "AlliGator Q Event in" {
    selector: "AlliGator Q Event in" -> [_ _ _ _ _ _ _ _ _ _ _ _ _ _ w348 _ _ _ _ w488 _ _]
    tunnel: "Data" -> [w31 w42 _ _ _ _ _ _ w130 w146 _ w190 w250 w303 _ w385 w394 w412 w441 w487 w526 _]
    tunnel: "AlliGator Q Elements" -> [w38 w51 w68 w78 w89 w99 w113 w120 w134 w140 w169 w176 w235 w288 w356 w387 w400 w406 w442 w489 w527 w531]
    tunnel: [w38 w50 w68 w78 w89 w99 w113 w120 w134 w139 w167 w175 w234 w287 w355 w387 w399 w405 w442 w489 w527 w531] -> w9
    tunnel: "VI in" -> [w28 _ w54 _ _ _ _ _ w127 _ w163 w185 w245 w297 w343 _ _ _ w426 w471 _ _]
    tunnel: w12 -> [w21 _ _ _ _ _ _ _ _ _ w172 _ _ _ _ _ _ _ w437 w477 _ _]
    tunnel: [w22 w46 w53 w74 w86 w98 w110 w119 w121 w137 w155 w194 w236 w305 w340 w386 w395 w403 w434 w474 w523 w530] -> w5
    tunnel: "Script in" -> [w22 w46 w53 w74 w86 w98 w110 w119 w121 w137 w155 w194 w236 w305 w340 w386 w395 w403 w434 w474 w523 w530]
    tunnel: "AlliGator" ("Sender") -> [_ _ _ _ _ _ _ _ _ _ _ _ _ _ _ w381 _ _ _ _ _ _]
    tunnel: w6 -> [w33 _ w58 _ _ _ _ _ w132 _ w170 w193 w252 w304 _ _ _ _ w433 w475 _ _]
    tunnel: "error in (no error)" -> [_ _ w59 w72 _ w93 _ w115 _ _ _ _ _ _ _ _ _ _ _ _ _ w529]
    tunnel: [w32 w40 w65 w75 w85 w95 w109 w116 w131 w136 w165 w195 w254 w307 w346 w379 w389 w402 w422 w476 w522 w529] -> w15
    tunnel: "AlliGator Ctrl Refnums" -> [w30 _ w64 _ w84 _ w108 _ w128 _ w162 w187 w246 w298 w344 w382 _ _ w431 w473 w521 _]
    tunnel: w17 -> [_ _ _ _ _ _ _ _ _ _ _ _ _ _ _ _ _ _ w432 w472 _ _]
    tunnel: "data value reference" -> [w27 w39 w62 w77 w82 w96 w106 w118 w126 w135 w157 w184 w243 w295 w342 w374 w388 w401 w425 w470 w518 w528]
    tunnel: [w25 w39 w61 w76 w81 w97 w105 w117 w124 w135 w157 w180 w244 w296 w342 w374 w388 w401 w423 w469 w517 w528] -> w7
    tunnel: [w23 _ "Phasor Calibration Map cleared." ("Message") w73 "Phasor Calibration Series cleared." ("Message") w94 "Phasor Calibration cleared." ("Message") w114 w122 _ w156 w177 w237 w289 w341 w373 _ _ w421 w468 w514 _] -> w3
    frame "Calibration:Apply Phasor Calibration" {
      # "\"Apply Phasor Calibration?\""
      n5 = call-poly "Variant to Data.vi"("Variant"=w31) -> ("Value"=w37:i32)  [unwired: 8 in]
      n6 = Unbundle By Name(w30) -> ("Registered Events Ctrl Refnums.Phasor Graph"=w36:refnum<vi>, "Phasor Graph Ctrl Refnums"=w29:T9)
      n7 = call "Show Animated Busy Icon with Message.vi"("Already active? (F)"=w22, "Message"=w33, "Target VI Refnum"=w28) -> ("Error Out"=w26:errorcluster)  [unwired: 8 in]
      n8 = call "AlliGator Apply Calibration Phasor(s) v2.vi"("Phasor Frequency"=w21, "Phasor Graph Ref"=w36, "Error In"=w26, "Plot Index (-1: last)"=w37, "Phasor Graph Ctrl Refnums"=w29, "AlliGator IV DVR"=w27) -> ("Error Out"=w34:errorcluster, "Calibrated Phasor"=w35:T25, "AlliGator IV DVR"=w25:refnum<data-value>, "Message"=w23:string)  [unwired: 1 in, 1 out]
      n9 = call "AlliGator Update Phasor Graph Information at Cursor.vi"("Valid?"=TRUE, "Error In"=w34, "Phasor"=w35, "Current Phasor Information Indicators"=w29) -> ("Error Out"=w24:errorcluster)  [unwired: 6 in, 1 out]
      n10 = call "Hide Animated Busy Icon with Message.vi"("Already active? (F)"=w22, "Error In"=w24, "Target VI reference"=w28) -> ("Error Out"=w32:errorcluster)  [unwired: 8 in]
    }
    frame "Calibration:Clear All Plots Calibrations" {
      w43 = -2147483648  # Selected Plots
      w44 = 2147483647  # All Plots
      # "\"Clear All Plots Calibrations\""
      n11 = call-poly "Variant to Data.vi"("Variant"=w42) -> ("Value"=w45:bool)  [unwired: 8 in]
      n12 = Select(t=w44, s=w45, f=w43) -> (s? t:f=w41:i32)
      n13 = Bundle By Name(cluster=T4 {"AlliGator Q Event"=enum."Calibration:Clear Plot(s) Calibration(s)?", "Data"=variant} ("Alligator Atomic Action"), "Data"=w41) -> (w48:T4)
      n14 = call-poly "AlliGator Add Action(s) to Stack.vi"("Elements Order in Action Stack (Default: 2 BEFORE 1)"=Alligator_Elements_Order_in_Action_Stack."Enqueue 2 BEFORE 1", "Alligator Atomic Action"=w48, "Alligator Queue Element 1"=w51) -> ("Error Out"=w40:errorcluster, "Alligator Queue Element 1 (+ 2)"=w50:T4[])  [unwired: 7 in]
    }
    frame "Calibration:Clear Calibration Map" {
      # "\"Clear Calibration Map\""
      n15 = Unbundle By Name(w64) -> ("Other AlliGator Ctrl Refnums.State Indicators"=w63:refnum<vi>)
      n16 = call "Show Animated Busy Icon with Message.vi"("Already active? (F)"=w53, "Message"=w58, "Error In"=w59, "Target VI Refnum"=w54) -> ("Error Out"=w57:errorcluster)  [unwired: 7 in]
      n17 = in-place {
        in-place-border: w57 -> [_]
        n18 = in-place-dvr #1(w62) -> (w70:T26)  [unwired: 1 out]
        n19 = in-place {
          n20 = in-place-cluster #2(w70) -> ()  [unwired: 1 out]
          n21 = in-place-cluster #2("Phasor Calibration Map"=T16 {"Phasor Frequency"=80000000.0, "Calibration Lifetime"=1e-09, "ROI Centers"=[], "ROI Descriptors"=[], "Map Resolution X"=0, "Map Resolution Y"=0, "z Array"=[]}) -> (w69:T26)
        }
        n22 = in-place-dvr #1(w69) -> (w61:refnum<data-value>, w56:errorcluster)
      }
      n23 = call "Hide Animated Busy Icon with Message.vi"("Already active? (F)"=w53, "Error In"=w56, "Target VI reference"=w54) -> ("Error Out"=w55:errorcluster)  [unwired: 8 in]
      n24 = call "AlliGator Get-Set State Indicators.vi"("State Indicators Refnum"=w63, "AlliGator State Indicators List"=AlliGator_State_Indicators_List."Phasor Calibration Map Defined" ("Time-Gated Phasor Analysis Task List"), "Error In"=w55, "ON/OFF"=FALSE ("Set (T)/Unset (F)"), "Set (T)/Get"=TRUE) -> ("Error Out"=w65:errorcluster)  [unwired: 8 in, 2 out]
    }
    frame "Calibration:Phasor Calibration Map Information" {
      # "\"Calibration:Phasor Calibration Map Information\""
      n25 = call "AlliGator Phasor Calibration Map Information.vi"("error in"=w72, "AlliGator IVDR"=w77) -> ("error out"=w75:errorcluster, "Message"=w73:string, "AlliGator IVDR"=w76:refnum<data-value>)  [unwired: 7 in]
    }
    frame "Calibration:Clear Calibration Series" {
      # "\"Clear Calibration Curve\""
      n26 = Unbundle By Name(w84) -> ("Other AlliGator Ctrl Refnums.State Indicators"=w83:refnum<vi>)
      n27 = in-place {
        n28 = in-place-dvr #3(w82) -> (w91:T26)  [unwired: 1 out]
        n29 = in-place {
          n30 = in-place-cluster #4(w91) -> ()  [unwired: 1 out]
          n31 = in-place-cluster #4("Calibration Phasor Series"=T18 {"m Array"=[], "phi Array"=[], "Phasor Frequency"=nan, "Calibration Lifetime"=nan} ("Phasor Reference Plot")) -> (w90:T26)
        }
        n32 = in-place-dvr #3(w90) -> (w81:refnum<data-value>)  [unwired: 1 out]
      }
      n33 = call "AlliGator Get-Set State Indicators.vi"("State Indicators Refnum"=w83, "AlliGator State Indicators List"=AlliGator_State_Indicators_List."Phasor Calibration Series Defined" ("Time-Gated Phasor Analysis Task List"), "ON/OFF"=FALSE ("Set (T)/Unset (F)"), "Set (T)/Get"=TRUE) -> ("Error Out"=w85:errorcluster)  [unwired: 9 in, 2 out]
    }
    frame "Calibration:Phasor Calibration Series Information" {
      # "\"Calibration:Phasor Calibration Series Information\""
      n34 = call "AlliGator Phasor Calibration Series Information.vi"("error in"=w93, "AlliGator IVDR"=w96) -> ("error out"=w95:errorcluster, "Message"=w94:string, "AlliGator IVDR"=w97:refnum<data-value>)  [unwired: 7 in]
    }
    frame "Calibration:Clear Phasor Calibration" {
      # "\"Clear Phasor Calibration\""
      n35 = Unbundle By Name(w108) -> ("Other AlliGator Ctrl Refnums.State Indicators"=w107:refnum<vi>)
      n36 = call "AlliGator IV Calibration Phasor.vi"("Get (F)/ Set (T)"=TRUE, "Calibration Phasor"=T19 {"m"=1.0, "phi"=0.0, "Phasor Frequency"=0.0, "Reference Lifetime"=0.0}, "AlliGator IV DVR in"=w106) -> ("error out"=w102:errorcluster, "AlliGator IV DVR out"=w105:refnum<data-value>)  [unwired: 6 in, 1 out]
      n37 = call "AlliGator Get-Set State Indicators.vi"("State Indicators Refnum"=w107, "AlliGator State Indicators List"=AlliGator_State_Indicators_List."Phasor Calibration Defined" ("Time-Gated Phasor Analysis Task List"), "Error In"=w102, "ON/OFF"=FALSE ("Set (T)/Unset (F)"), "Set (T)/Get"=TRUE) -> ("Error Out"=w109:errorcluster)  [unwired: 8 in, 2 out]
    }
    frame "Calibration:Single Phasor Calibration Information" {
      # "\"Calibration:Single Phasor Calibration Information\""
      n38 = call "AlliGator Single Phasor Calibration Information.vi"("error in"=w115, "AlliGator IVDR"=w118) -> ("error out"=w116:errorcluster, "Message"=w114:string, "AlliGator IVDR"=w117:refnum<data-value>)  [unwired: 7 in]
    }
    frame "Calibration:Clear Plot(s) Calibration(s)?" {
      # "\"Clear Plot(s) Calibration(s)?\""
      n39 = Unbundle By Name(w128) -> ("Registered Events Ctrl Refnums.Phasor Graph"=w133:refnum<vi>)
      n40 = call-poly "Variant to Data.vi"("Variant"=w130) -> ("Value"=w129:i32)  [unwired: 8 in]
      n41 = call "Show Animated Busy Icon with Message.vi"("Already active? (F)"=w121, "Message"=w132, "Target VI Refnum"=w127) -> ("Error Out"=w125:errorcluster)  [unwired: 8 in]
      n42 = call "AlliGator Clear Plot(s) Calibration(s).vi"("Phasor Graph Ref"=w133, "Error In"=w125, "Plot Index (-1: last)"=w129, "AlliGator IV DVR"=w126) -> ("Error Out"=w123:errorcluster, "Message"=w122:string, "AlliGator IV DVR"=w124:refnum<data-value>)  [unwired: 4 in, 1 out]
      n43 = call "Hide Animated Busy Icon with Message.vi"("Already active? (F)"=w121, "Error In"=w123, "Target VI reference"=w127) -> ("Error Out"=w131:errorcluster)  [unwired: 8 in]
    }
    frame "Calibration:Clear Single Plot Calibration" {
      # "\"Clear Single Plot Calibration\""
      n44 = Variant To Data(type=T20 {"Multiplot XY Graph"=refnum, "Mouse Coordinates"={"Horizontal"=0, "Vertical"=0}} ("Mouse Click Event Data"), Variant=w146) -> (data=w144:T20, error out=w141:errorcluster)  [unwired: 1 in]
      n45 = Unbundle(w144) -> ("Multiplot XY Graph"=w143:T21, "Mouse Coordinates"=w142:T22)
      n46 = call-poly "Get Plot at Mouse Click.vi"("error in (no error)"=w141, "Mouse Click Coordinates"=w142, "XYGraph Ref"=w143) -> ("error out"=w136:errorcluster, "Plot at Coordinates"=w138:i32)  [unwired: 2 in, 5 out]
      n47 = case shown="1, Default" w138 {
        selector: w138 -> [_ w148]
        tunnel: w140 -> [w147 w154]
        tunnel: [w147 w153] -> w139
        tunnel: w136 -> [_ w152]
        frame 0 {
          # "The first plot is the UC"
        }
        frame 1, Default {
          n48 = Bundle By Name(cluster=T4 {"AlliGator Q Event"=enum."Calibration:Clear Plot(s) Calibration(s)?", "Data"=variant} ("Alligator Atomic Action"), "Data"=w148) -> (w150:T4)
          n49 = call-poly "AlliGator Add Action(s) to Stack.vi"("Elements Order in Action Stack (Default: 2 BEFORE 1)"=Alligator_Elements_Order_in_Action_Stack."Enqueue 2 BEFORE 1", "Error In"=w152, "Alligator Atomic Action"=w150, "Alligator Queue Element 1"=w154) -> ("Alligator Queue Element 1 (+ 2)"=w153:T4[])  [unwired: 6 in, 1 out]
        }
      }
    }
    frame "Calibration:Compute Optimal Calibration from Phasor References" {
      # "\"Compute Optimal Calibration from Phasor References\""
      n50 = Unbundle By Name(w162) -> ("Phasor Graph Ctrl Refnums.Calibration Lifetime"=w161:refnum<vi>)
      n51 = call "Show Animated Busy Icon with Message.vi"("Already active? (F)"=w155, "Message"=w170, "Target VI Refnum"=w163) -> ("Error Out"=w171:errorcluster)  [unwired: 8 in]
      n52 = call "AlliGator Find Optimal Phasor Calibration (no Starting Calibration).vi"("Error In"=w171, "Phasor Frequency"=w172) -> ("Error Out"=w159:errorcluster, "tau 2"=w173:dbl[unit], "tau 1"=w160:dbl[unit], "Calibration Phasor (g, s)"=w174:T25, "Message"=w156:string)  [unwired: 5 in]
      n53 = property class="DigNum (strict)"(reference=w161, error in=w159, "Val(Sgnl)"=w160) -> (error out=w158:errorcluster)  [unwired: 1 out]
      n54 = call "AlliGator Update Phasor Calibration & References.vi"("tau 2"=w173, "tau 1"=w160, "error in (no error)"=w158, "Calibration Phasor"=w174) -> ("Error Out"=w166:errorcluster, "Named Q Element out"=w168:T4[])  [unwired: 6 in]
      n55 = call-poly "AlliGator Add Action(s) to Stack.vi"("Elements Order in Action Stack (Default: 2 BEFORE 1)"=Alligator_Elements_Order_in_Action_Stack."Enqueue 2 BEFORE 1", "Error In"=w166, "Alligator Queue Element 2"=w168, "Alligator Queue Element 1"=w169) -> ("Error Out"=w165:errorcluster, "Alligator Queue Element 1 (+ 2)"=w167:T4[])  [unwired: 6 in]
    }
    frame "Calibration:Load/Save Phasor Calibration Map" {
      # "\"Load/Save Phasor Calibration Map\""
      n56 = Variant To Data(type=T23 {"Load/Save"=FALSE, "File Path"=path ""}, Variant=w190) -> (data=w192:T23, error out=w183:errorcluster)  [unwired: 1 in]
      n57 = Unbundle By Name(w187) -> ("Other AlliGator Ctrl Refnums.State Indicators"=w186:refnum<vi>)
      n58 = Unbundle By Name(w192) -> ("File Path"=w188:path, "Load/Save"=w189:bool)
      n59 = call "AlliGator IV Calibration Phasor Map.vi"("Get (F)/ Set (T)"=FALSE, "error in (no error)"=w183, "AlliGator IV DVR in"=w184) -> ("error out"=w179:errorcluster, "Phasor Calibration Map"=w182:T16, "AlliGator IV DVR out"=w181:refnum<data-value>)  [unwired: 6 in]
      n60 = case shown="False" w189 {
        tunnel: w186 -> [w219 _]
        tunnel: [w199 w225] -> w195
        tunnel: w194 -> [w207 w223]
        tunnel: w193 -> [w217 w226]
        tunnel: w188 -> [w209 w229]
        tunnel: w185 -> [w208 w224]
        tunnel: w182 -> [w216 w232]
        tunnel: w181 -> [w215 w230]
        tunnel: [w214 w230] -> w180
        tunnel: w179 -> [w211 w231]
        tunnel: [w198 w228] -> w177
        tunnel: w176 -> [w202 w222]
        tunnel: [w201 w222] -> w175
        frame False {
          w196 = TRUE ("Set (T)/Unset (F)")
          # "Load"
          n61 = call "Show Animated Busy Icon with Message.vi"("Already active? (F)"=w207, "Message"=w217, "Error In"=w211, "Target VI Refnum"=w208) -> ("Error Out"=w218:errorcluster)  [unwired: 7 in]
          n62 = call "AlliGator Load Calibration Phasor Map.vi"("Error In"=w218, "File Path (empty: dialog)"=w209, "Calibration Phasor Map in"=w216) -> ("error out"=w220:errorcluster, "Phasor Frequency"=w197:dbl[unit], "Calibration Phasor Map out"=w212:T16, "Message"=w198:string)  [unwired: 4 in, 1 out]
          n63 = call "Hide Animated Busy Icon with Message.vi"("Already active? (F)"=w207, "Error In"=w220, "Target VI reference"=w208) -> ("Error Out"=w213:errorcluster)  [unwired: 8 in]
          n64 = call "AlliGator IV Calibration Phasor Map.vi"("Get (F)/ Set (T)"=TRUE, "error in (no error)"=w213, "Phasor Calibration Map 2"=w212, "AlliGator IV DVR in"=w215) -> ("error out"=w206:errorcluster, "AlliGator IV DVR out"=w214:refnum<data-value>)  [unwired: 5 in, 1 out]
          n65 = call "AlliGator Get-Set State Indicators.vi"("State Indicators Refnum"=w219, "AlliGator State Indicators List"=AlliGator_State_Indicators_List."Phasor Calibration Map Defined" ("Time-Gated Phasor Analysis Task List"), "Error In"=w206, "ON/OFF"=w196, "Set (T)/Get"=w196) -> ("Error Out"=w200:errorcluster)  [unwired: 8 in, 2 out]
          n66 = Bundle By Name(cluster=T4 {"AlliGator Q Event"=enum."GUI:Set Phasor Frequency", "Data"=variant} ("Alligator Atomic Action"), "Data"=w197) -> (w203:T4)
          n67 = call-poly "AlliGator Add Action(s) to Stack.vi"("Elements Order in Action Stack (Default: 2 BEFORE 1)"=Alligator_Elements_Order_in_Action_Stack."Enqueue 2 BEFORE 1", "Error In"=w200, "Alligator Atomic Action"=w203, "Alligator Queue Element 1"=w202) -> ("Error Out"=w199:errorcluster, "Alligator Queue Element 1 (+ 2)"=w201:T4[])  [unwired: 6 in]
        }
        frame True {
          # "Save"
          n68 = call "Show Animated Busy Icon with Message.vi"("Already active? (F)"=w223, "Message"=w226, "Error In"=w231, "Target VI Refnum"=w224) -> ("Error Out"=w227:errorcluster)  [unwired: 7 in]
          n69 = call "AlliGator Save Calibration Phasor Map.vi"("Error In"=w227, "File Path (empty: dialog)"=w229, "Calibration Phasor Map"=w232) -> ("error out"=w233:errorcluster, "Message"=w228:string)  [unwired: 6 in, 1 out]
          n70 = call "Hide Animated Busy Icon with Message.vi"("Already active? (F)"=w223, "Error In"=w233, "Target VI reference"=w224) -> ("Error Out"=w225:errorcluster)  [unwired: 8 in]
        }
      }
    }
    frame "Calibration:Load/Save Phasor Calibration Series" {
      # "\"Load/Save Phasor Calibration Series\""
      n71 = Variant To Data(type=T23 {"Load/Save"=FALSE, "File Path"=path ""}, Variant=w250) -> (data=w251:T23, error out=w242:errorcluster)  [unwired: 1 in]
      n72 = Unbundle By Name(w246) -> ("Other AlliGator Ctrl Refnums.State Indicators"=w253:refnum<vi>)
      n73 = Unbundle By Name(w251) -> ("File Path"=w247:path, "Load/Save"=w248:bool)
      n74 = call "AlliGator IV Calibration Phasor Series.vi"("Get (F)/ Set (T)"=FALSE, "error in (no error)"=w242, "AlliGator IV DVR in"=w243) -> ("error out"=w240:errorcluster, "Calibration Phasor Series"=w238:T18, "AlliGator IV DVR out"=w241:refnum<data-value>)  [unwired: 6 in]
      n75 = case shown="False" w248 {
        tunnel: [w258 w286] -> w254
        tunnel: w253 -> [w278 _]
        tunnel: w252 -> [w276 _]
        tunnel: w247 -> [w267 _]
        tunnel: w240 -> [w274 w284]
        tunnel: w245 -> [w275 _]
        tunnel: w241 -> [w273 w285]
        tunnel: [w272 w285] -> w244
        tunnel: w238 -> [w268 w283]
        tunnel: [w256 w282] -> w237
        tunnel: w236 -> [w265 _]
        tunnel: w235 -> [w261 w281]
        tunnel: [w260 w281] -> w234
        frame False {
          w255 = TRUE ("Set (T)/Unset (F)")
          # "Load"
          n76 = call "Show Animated Busy Icon with Message.vi"("Already active? (F)"=w265, "Message"=w276, "Error In"=w274, "Target VI Refnum"=w275) -> ("Error Out"=w277:errorcluster)  [unwired: 7 in]
          n77 = call "AlliGator Load Calibration Phasor Series.vi"("Error In"=w277, "File Path"=w267, "Calibration Phasor Series in"=w268) -> ("error out"=w279:errorcluster, "Phasor Frequency"=w257:dbl[unit], "Calibration Phasor Series out"=w270:T18, "Message"=w256:string)  [unwired: 4 in, 1 out]
          n78 = call "Hide Animated Busy Icon with Message.vi"("Already active? (F)"=w265, "Error In"=w279, "Target VI reference"=w275) -> ("Error Out"=w271:errorcluster)  [unwired: 8 in]
          n79 = call "AlliGator IV Calibration Phasor Series.vi"("Get (F)/ Set (T)"=TRUE, "error in (no error)"=w271, "Calibration Phasor Series"=w270, "AlliGator IV DVR in"=w273) -> ("error out"=w266:errorcluster, "AlliGator IV DVR out"=w272:refnum<data-value>)  [unwired: 5 in, 1 out]
          n80 = call "AlliGator Get-Set State Indicators.vi"("State Indicators Refnum"=w278, "AlliGator State Indicators List"=AlliGator_State_Indicators_List."Phasor Calibration Series Defined" ("Time-Gated Phasor Analysis Task List"), "Error In"=w266, "ON/OFF"=w255, "Set (T)/Get"=w255) -> ("Error Out"=w259:errorcluster)  [unwired: 8 in, 2 out]
          n81 = Bundle By Name(cluster=T4 {"AlliGator Q Event"=enum."GUI:Set Phasor Frequency", "Data"=variant} ("Alligator Atomic Action"), "Data"=w257) -> (w262:T4)
          n82 = call-poly "AlliGator Add Action(s) to Stack.vi"("Elements Order in Action Stack (Default: 2 BEFORE 1)"=Alligator_Elements_Order_in_Action_Stack."Enqueue 2 BEFORE 1", "Error In"=w259, "Alligator Atomic Action"=w262, "Alligator Queue Element 1"=w261) -> ("Error Out"=w258:errorcluster, "Alligator Queue Element 1 (+ 2)"=w260:T4[])  [unwired: 6 in]
        }
        frame True {
          # "Save"
          n83 = call "AlliGator Save Calibration Phasor Series.vi"("Error In"=w284, "Calibration Phasor Series"=w283) -> ("error out"=w286:errorcluster, "Message"=w282:string)  [unwired: 7 in, 1 out]
        }
      }
    }
    frame "Calibration:Load/Save Phasor Calibration" {
      # "\"Load/Save Phasor Calibration\""
      n84 = Variant To Data(type=T23 {"Load/Save"=FALSE, "File Path"=path ""}, Variant=w303) -> (data=w301:T23, error out=w294:errorcluster)  [unwired: 1 in]
      n85 = Unbundle By Name(w301) -> ("File Path"=w299:path, "Load/Save"=w300:bool)
      n86 = Unbundle By Name(w298) -> ("Other AlliGator Ctrl Refnums.State Indicators"=w306:refnum<vi>)
      n87 = call "AlliGator IV Calibration Phasor.vi"("Get (F)/ Set (T)"=FALSE, "error in (no error)"=w294, "AlliGator IV DVR in"=w295) -> ("error out"=w292:errorcluster, "Calibration Phasor"=w290:T19, "AlliGator IV DVR out"=w293:refnum<data-value>)  [unwired: 6 in]
      n88 = case shown="False" w300 {
        tunnel: w306 -> [w332 _]
        tunnel: [w309 w339] -> w307
        tunnel: w305 -> [w319 _]
        tunnel: w304 -> [w329 _]
        tunnel: w299 -> [w321 _]
        tunnel: w292 -> [w324 w337]
        tunnel: w297 -> [w328 _]
        tunnel: w293 -> [w327 w338]
        tunnel: [w325 w338] -> w296
        tunnel: w290 -> [w322 w336]
        tunnel: [w320 w335] -> w289
        tunnel: w288 -> [w318 w334]
        tunnel: [w313 w334] -> w287
        frame False {
          w308 = TRUE ("Set (T)/Unset (F)")
          # "Load"
          n89 = call "Show Animated Busy Icon with Message.vi"("Already active? (F)"=w319, "Message"=w329, "Error In"=w324, "Target VI Refnum"=w328) -> ("Error Out"=w330:errorcluster)  [unwired: 7 in]
          n90 = call "AlliGator Load Calibration Phasor.vi"("Error In"=w330, "File Path"=w321, "Calibration Phasor in"=w322) -> ("error out"=w331:errorcluster, "Phasor Frequency"=w315:dbl[unit], "Calibration Phasor out"=w326:T19, "Message"=w320:string)  [unwired: 4 in, 1 out]
          n91 = call "Hide Animated Busy Icon with Message and Abort Button.vi"("Already active? (F)"=w319, "Target VI reference"=w328, "Error In"=w331) -> ("Error Out"=w312:errorcluster)  [unwired: 16 in]
          n92 = Bundle By Name(cluster=T4 {"AlliGator Q Event"=enum."GUI:Set Phasor Frequency", "Data"=variant} ("Alligator Atomic Action"), "Data"=w315) -> (w314:T4)
          n93 = call "AlliGator IV Calibration Phasor.vi"("Get (F)/ Set (T)"=TRUE, "error in (no error)"=w312, "Calibration Phasor"=w326, "AlliGator IV DVR in"=w327) -> ("error out"=w311:errorcluster, "AlliGator IV DVR out"=w325:refnum<data-value>)  [unwired: 5 in, 1 out]
          n94 = call "AlliGator Get-Set State Indicators.vi"("State Indicators Refnum"=w332, "AlliGator State Indicators List"=AlliGator_State_Indicators_List."Phasor Calibration Defined" ("Time-Gated Phasor Analysis Task List"), "Error In"=w311, "ON/OFF"=w308, "Set (T)/Get"=w308) -> ("Error Out"=w310:errorcluster)  [unwired: 8 in, 2 out]
          n95 = call-poly "AlliGator Add Action(s) to Stack.vi"("Elements Order in Action Stack (Default: 2 BEFORE 1)"=Alligator_Elements_Order_in_Action_Stack."Enqueue 2 BEFORE 1", "Error In"=w310, "Alligator Atomic Action"=w314, "Alligator Queue Element 1"=w318) -> ("Error Out"=w309:errorcluster, "Alligator Queue Element 1 (+ 2)"=w313:T4[])  [unwired: 6 in]
        }
        frame True {
          # "Save"
          n96 = call "AlliGator Save Calibration Phasor.vi"("Error In"=w337, "Calibration Phasor"=w336) -> ("error out"=w339:errorcluster, "Message"=w335:string)  [unwired: 7 in, 1 out]
        }
      }
    }
    frame "Calibration:Phasor Calibration Maps (# Gates Series)" {
      # "\"Phasor Calibration Maps (# Gates Series)\""
      n97 = Unbundle By Name(w344) -> ("Registered Events Ctrl Refnums.Phasor Graph"=w345:refnum<vi>)
      n98 = call "Enum to String.vim"("Enum"=w348) -> ("String"=w347:string)
      n99 = call "AlliGator Phasor Calibration Map Series Dialog.vi"() -> ("File Name (# Steps will be added)"=w354:string, "Destination Folder"=w353:path, "Gate Step Series"=w352:string, "Phasor Calibration Dataset Path"=w351:path, "OK"=w349:bool, "error out"=w350:errorcluster)  [unwired: 14 in]
      n100 = case shown="True" w349 {
        tunnel: w356 -> [w358 w372]
        tunnel: [w358 w371] -> w355
        tunnel: w354 -> [_ w370]
        tunnel: w353 -> [_ w369]
        tunnel: w352 -> [_ w368]
        tunnel: w351 -> [_ w367]
        tunnel: w350 -> [w357 w366]
        tunnel: w345 -> [_ w365]
        tunnel: w340 -> [_ w359]
        tunnel: w347 -> [_ w364]
        tunnel: [w357 w363] -> w346
        tunnel: w343 -> [_ w361]
        tunnel: [_ w360] -> w341
        frame False {
        }
        frame True {
          n101 = call "AlliGator Phasor Calibration Maps (# Gates Series) Script.vi"("Alligator Queue Elements in"=w372, "Phasor Graph refnum"=w365, "File Name (# Steps will be added)"=w370, "Destination Folder"=w369, "Gate Step Series"=w368, "Error In"=w366, "Phasor Calibration Dataset Path"=w367) -> ("Alligator Queue Elements out"=w371:T4[], "Message"=w360:string, "Error Out"=w362:errorcluster)  [unwired: 6 in]
          n102 = call "Show Animated Busy Icon with Message and Abort Button.vi"("Already active? (F)"=w359, "Message"=w364, "Target VI reference"=w361, "Error In"=w362) -> ("Error Out"=w363:errorcluster)  [unwired: 15 in]
        }
      }
    }
    frame "Calibration:Set Calibration Type" {
      # "\"Calibration:Set Calibration Type\""
      n103 = Variant To Data(type=Phasor_Calibration_Type."None" ("Calibration Type"), Variant=w385) -> (data=w375:T24, error out=w383:errorcluster)  [unwired: 1 in]
      n104 = Unbundle By Name(w382) -> ("Phasor Graph Ctrl Refnums.Calibration Type"=w376:refnum<vi>, "Other AlliGator Ctrl Refnums.State Indicators"=w380:refnum<vi>)
      n105 = call "AlliGator Update Settings & Control.vi"("Error In"=w383, "Value"=w375, "Sender"=w381, "CtlRef"=w376) -> ("Error Out"=w378:errorcluster)  [unwired: 7 in]
      n106 = property class="Enum (strict)"(reference=w376, error in=w378, "Value"=w375) -> (error out=w377:errorcluster)  [unwired: 1 out]
      n107 = call "AlliGator Set Calibration Type Status LEDs.vi"("error in (no error)"=w377, "Calibration Type"=w375, "State Indicators"=w380) -> ("error out"=w379:errorcluster, "Message"=w373:string)  [unwired: 7 in]
    }
    frame "Calibration:Update Multiple Plots Calibration" {
      w390 = -2147483648  # Selected Plots: -2^31
      w392 = 2147483647  # All Plots: 2^31-1
      # "\"Update All Plots Calibrations\""
      n108 = call-poly "Variant to Data.vi"("Variant"=w394) -> ("Value"=w393:bool)  [unwired: 8 in]
      n109 = Select(t=w392, s=w393, f=w390) -> (s? t:f=w391:i32)
      n110 = Bundle By Name(cluster=T4 {"AlliGator Q Event"=enum."Calibration:Apply Phasor Calibration", "Data"=variant} ("Alligator Atomic Action"), "Data"=w391) -> (w397:T4)
      n111 = call-poly "AlliGator Add Action(s) to Stack.vi"("Elements Order in Action Stack (Default: 2 BEFORE 1)"=Alligator_Elements_Order_in_Action_Stack."Enqueue 2 BEFORE 1", "Alligator Atomic Action"=w397, "Alligator Queue Element 1"=w400) -> ("Error Out"=w389:errorcluster, "Alligator Queue Element 1 (+ 2)"=w399:T4[])  [unwired: 7 in]
    }
    frame "Calibration:Update Single Plot Calibration" {
      # "\"Update Single Plot Calibration\""
      n112 = Variant To Data(type=T20 {"Multiplot XY Graph"=refnum, "Mouse Coordinates"={"Horizontal"=0, "Vertical"=0}} ("Mouse Click Event Data"), Variant=w412) -> (data=w410:T20, error out=w407:errorcluster)  [unwired: 1 in]
      n113 = Unbundle(w410) -> ("Multiplot XY Graph"=w409:T21, "Mouse Coordinates"=w408:T22)
      n114 = call-poly "Get Plot at Mouse Click.vi"("error in (no error)"=w407, "Mouse Click Coordinates"=w408, "XYGraph Ref"=w409) -> ("error out"=w402:errorcluster, "Plot at Coordinates"=w404:i32)  [unwired: 2 in, 5 out]
      n115 = case shown="1, Default" w404 {
        selector: w404 -> [_ w414]
        tunnel: w406 -> [w413 w420]
        tunnel: [w413 w419] -> w405
        tunnel: w402 -> [_ w418]
        frame 0 {
          # "The first plot is the UC"
        }
        frame 1, Default {
          n116 = Bundle By Name(cluster=T4 {"AlliGator Q Event"=enum."Calibration:Apply Phasor Calibration", "Data"=variant} ("Alligator Atomic Action"), "Data"=w414) -> (w416:T4)
          n117 = call-poly "AlliGator Add Action(s) to Stack.vi"("Elements Order in Action Stack (Default: 2 BEFORE 1)"=Alligator_Elements_Order_in_Action_Stack."Enqueue 2 BEFORE 1", "Error In"=w418, "Alligator Atomic Action"=w416, "Alligator Queue Element 1"=w420) -> ("Alligator Queue Element 1 (+ 2)"=w419:T4[])  [unwired: 6 in, 1 out]
        }
      }
    }
    frame "Calibration:Use as Calibration Map" {
      # "\"Use as Calibration Map\""
      n118 = Unbundle By Name(w431) -> ("Other AlliGator Ctrl Refnums.State Indicators"=w435:refnum<vi>)
      n119 = Variant To Data(type=T20 {"Multiplot XY Graph"=refnum, "Mouse Coordinates"={"Horizontal"=0, "Vertical"=0}} ("Mouse Click Event Data"), Variant=w441) -> (data=w429:T20, error out=w436:errorcluster)  [unwired: 1 in]
      n120 = Unbundle(w429) -> ("Multiplot XY Graph"=w428:T21, "Mouse Coordinates"=w427:T22)
      n121 = call-poly "Get Plot at Mouse Click.vi"("error in (no error)"=w436, "Mouse Click Coordinates"=w427, "XYGraph Ref"=w428) -> ("error out"=w424:errorcluster, "Plot at Coordinates"=w439:i32, "XYGraph Ref"=w440:T21, "Plot Name"=w438:string)  [unwired: 2 in, 3 out]
      n122 = case shown="1, Default" w439 {
        selector: w439 -> [_ w453]
        tunnel: w437 -> [_ w461]
        tunnel: w440 -> [_ _]
        tunnel: w432 -> [_ w460]
        tunnel: w438 -> [_ w458]
        tunnel: w424 -> [w443 w459]
        tunnel: w435 -> [_ w456]
        tunnel: w434 -> [_ w447]
        tunnel: w433 -> [_ w454]
        tunnel: w426 -> [_ w452]
        tunnel: w425 -> [w444 w451]
        tunnel: [w444 w450] -> w423
        tunnel: [w443 w449] -> w422
        tunnel: [_ w448] -> w421
        frame 0 {
          # "UC or SEPL"
        }
        frame 1, Default {
          n123 = call "Show Animated Busy Icon with Message.vi"("Already active? (F)"=w447, "Message"=w454, "Error In"=w459, "Target VI Refnum"=w452) -> ("Error Out"=w455:errorcluster)  [unwired: 7 in]
          n124 = call "AlliGator Use Phasor Plot as Phasor Calibration Map.vi"("Calibration Lifetime"=w460, "Phasor Frequency"=w461, "error in (no error)"=w455, "Plot Name"=w458, "Phasor Graph Plot index"=w453, "Data Value Reference in"=w451) -> ("error out"=w446:errorcluster, "Message"=w448:string, "Valid Map?"=w457:bool, "Data Value Reference out"=w450:refnum<data-value>)  [unwired: 2 in]
          n125 = case shown="True" w457 {
            tunnel: w456 -> [_ w466]
            tunnel: w446 -> [w462 w465]
            tunnel: [w462 w464] -> w445
            frame False {
              n126 = call "Play Error Sound.vi"() -> ()  [unwired: 27 in, 1 out]
            }
            frame True {
              w463 = TRUE ("Set (T)/Unset (F)")
              n127 = call "AlliGator Get-Set State Indicators.vi"("State Indicators Refnum"=w466, "AlliGator State Indicators List"=AlliGator_State_Indicators_List."Phasor Calibration Map Defined" ("Time-Gated Phasor Analysis Task List"), "Error In"=w465, "ON/OFF"=w463, "Set (T)/Get"=w463) -> ("Error Out"=w464:errorcluster)  [unwired: 8 in, 2 out]
            }
          }
          n128 = call "Hide Animated Busy Icon with Message.vi"("Already active? (F)"=w447, "Error In"=w445, "Target VI reference"=w452) -> ("Error Out"=w449:errorcluster)  [unwired: 8 in]
        }
      }
    }
    frame "Calibration:Use as Calibration Series" {
      # "\"Use as Calibration Series\""
      n129 = Variant To Data(type=T20 {"Multiplot XY Graph"=refnum, "Mouse Coordinates"={"Horizontal"=0, "Vertical"=0}} ("Mouse Click Event Data"), Variant=w487) -> (data=w485:T20, error out=w482:errorcluster)  [unwired: 1 in]
      n130 = Unbundle(w485) -> ("Multiplot XY Graph"=w484:T21, "Mouse Coordinates"=w483:T22)
      n131 = call-poly "Get Plot at Mouse Click.vi"("error in (no error)"=w482, "Mouse Click Coordinates"=w483, "XYGraph Ref"=w484) -> ("error out"=w481:errorcluster, "Plot at Coordinates"=w479:i32, "XYGraph Ref"=w480:T21, "Plot Name"=w478:string)  [unwired: 2 in, 3 out]
      n132 = case shown="1, Default" w479 {
        selector: w479 -> [_ w509]
        tunnel: w488 -> [_ w512]
        tunnel: w477 -> [_ w511]
        tunnel: w481 -> [w490 w510]
        tunnel: w480 -> [_ _]
        tunnel: w472 -> [_ w507]
        tunnel: w470 -> [w491 w506]
        tunnel: [w491 w505] -> w469
        tunnel: w478 -> [_ w504]
        tunnel: [w490 w494] -> w476
        tunnel: w475 -> [_ w500]
        tunnel: w474 -> [_ w493]
        tunnel: w473 -> [_ w498]
        tunnel: w471 -> [_ w496]
        tunnel: [_ w495] -> w468
        frame ..0 {
          # "not found (<0) or UC (0)"
        }
        frame 1, Default {
          w492 = TRUE ("Set (T)/Unset (F)")
          n133 = call "Show Animated Busy Icon with Message.vi"("Already active? (F)"=w493, "Message"=w500, "Error In"=w510, "Target VI Refnum"=w496) -> ("Error Out"=w501:errorcluster)  [unwired: 7 in]
          n134 = Unbundle By Name(w498) -> ("Other AlliGator Ctrl Refnums.State Indicators"=w497:refnum<vi>)
          n135 = call "AlliGator Use Phasor Plot as Phasor Calibration Series.vi"("Calibration Lifetime"=w507, "Phasor Frequency"=w511, "error in (no error)"=w501, "Phasor Graph Plot index"=w509, "Data Value Reference in"=w506) -> ("error out"=w502:errorcluster, "Data Value Reference out"=w505:refnum<data-value>)  [unwired: 5 in]
          n136 = call "Hide Animated Busy Icon with Message.vi"("Already active? (F)"=w493, "Error In"=w502, "Target VI reference"=w496) -> ("Error Out"=w499:errorcluster)  [unwired: 8 in]
          n137 = Format Into String(format string="%s: %s", error in=w499, w512, w504) -> (resulting string=w495:string, error out=w494:errorcluster)  [unwired: 1 in]
          n138 = call "AlliGator Get-Set State Indicators.vi"("State Indicators Refnum"=w497, "AlliGator State Indicators List"=AlliGator_State_Indicators_List."Phasor Calibration Series Defined" ("Time-Gated Phasor Analysis Task List"), "Error In"=w499, "ON/OFF"=w492, "Set (T)/Get"=w492) -> ()  [unwired: 8 in, 3 out]
        }
      }
    }
    frame "Calibration:Use as Calibration" {
      w513 = TRUE ("Set (T)/Unset (F)")
      # "\"Use as Calibration\""
      n139 = Unbundle By Name(w521) -> ("Other AlliGator Ctrl Refnums.State Indicators"=w520:refnum<vi>)
      n140 = Variant To Data(type=T25 {"g"=0.0, "s"=0.0} ("Phasor (g, s)"), Variant=w526) -> (data=w515:T25, error out=w524:errorcluster)  [unwired: 1 in]
      n141 = Unbundle By Name(w524) -> ("status"=w516:bool)
      n142 = call "AlliGator Update IV Calibration Phasor.vi"("Phasor"=w515, "Use Last Raw Phasor"=w516, "AlliGator IV DVR in"=w518) -> ("error out"=w522:errorcluster, "Message"=w514:string, "AlliGator IV DVR out"=w517:refnum<data-value>)  [unwired: 6 in]
      n143 = call "AlliGator Get-Set State Indicators.vi"("State Indicators Refnum"=w520, "AlliGator State Indicators List"=AlliGator_State_Indicators_List."Phasor Calibration Defined" ("Time-Gated Phasor Analysis Task List"), "ON/OFF"=w513, "Set (T)/Get"=w513) -> ()  [unwired: 9 in, 3 out]
    }
    frame Default {
      # "\"---- Phasor Calibration ----\""
    }
  }
  "error out" <- w15
  "Alligator Queue Element 1 (+ 2)" <- w9
  "AlliGator IV DVR" <- w7
  "Script out" <- w5
  n144 = call "Message Style.vi"() -> ("Message Formatting"=w2:T2)
  n145 = call "AlliGator Package Notebook Messages.vi"("Message Formatting"=w2, "Message"=w3, "AlliGator Q Event in"="AlliGator Q Event in") -> ("[Notebook Message]"=→"[Notebook Message]":T1[])  [unwired: 8 in]
